vi "信号光谱8.vi"() -> ()   [LabVIEW 2018]
uses:
  <vilib>/Utility/NIReport.llb/Report Type.ctl
  <vilib>/Utility/file.llb/Write Delimited Spreadsheet (DBL).vi
  <vilib>/Instr/_visa.llb/VISA Configure Serial Port (Instr).vi
  <vilib>/addons/_office/excel.llb/Excel Get Data ([str]).vi
  <vilib>/Utility/NIReport.llb/NI_report.lvclass
  <vilib>/Analysis/NI_AALBase.lvlib
  <vilib>/ptbypt/NI_PtbyPt.lvlib
  <vilib>/Utility/NIReport.llb/NI_ReportGenerationCore.lvlib
  <vilib>/addons/_office/NI_ReportGenerationToolkit.lvlib
  <vilib>/Utility/NIReport.llb/Excel/NI_Excel.lvclass
panel:
  in  "上升下降沿/s":dbl format="%.2p"
  in  "延时/s":dbl format="%.2p"
  in  "占空比/%":dbl=3.0 format="%.2p"
  in  "高电平/V":dbl=4.0 format="%.2p"
  in  "频率/Hz":dbl=6000.0 format="%.3p"
  in  "低电平/V":dbl min=0.0 max=5.0 format="%.2p"
  in  "Enable":bool
  in  "上升下降沿":i32(ring)=1 items=["上升沿", "下降沿"]
  in  "输出信号波形":u16(ring) items=["Pulse"]
  out "Output":bool
  in  "VISA 信号发生器":refnum<visa-resource-name>="USB0::0x1AB1::0x0641::DG4E192200870::INSTR"
  out "Output 2":bool
  in  "Enable 2":bool
  in  "上升下降沿/s 2":dbl format="%.2p"
  in  "延时/s 2":dbl format="%.2p"
  in  "占空比/% 2":dbl=3.0 format="%.2p"
  in  "高电平/V 2":dbl=0.002 format="%.2p"
  in  "频率/Hz 2":dbl=6000.0 format="%.3p"
  in  "低电平/V 2":dbl min=0.0 max=5.0 format="%.2p"
  in  "上升下降沿 2":i32(ring)=1 items=["上升沿", "下降沿"]
  in  "输出信号波形 2":u16(ring) items=["Pulse"]
  in  "终止测量":bool
  in  "测量次数":i32=1
  out "best fit":cluster{"Y":dbl[], "Y":dbl[]}[](graph)
  in  "拟合终点":i32=700
  in  "拟合起点":i32=350
  out "angle":dbl
  out "图片地址":string
  in  "开光时间/ms":u32=50
  out "最终存储路径 2":path
  out "照明光error out":errorcluster
  in  "照明光":bool
  in  "stop bits (10: 1 bit)":u16(ring)=10 items=["1.0"=10, "1.5"=15, "2.0"=20]
  in  "parity (0:none)":enum16{"None", "Odd", "Even", "Mark", "Space"}(ring)
  in  "data bits (8)":u16=8 min=5 max=8 step=1
  in  "baud rate":u32=9600 caption="baud rate (115200)" min=9600 max=115200
  in  "照明光VISA":refnum<visa-resource-name>="COM7"
  out "正在测量":bool
  in  "滤波阈值":dbl=1500.0 format="%#_13g"
  out "范围内？":bool[](array[boolean])
  out "w":dbl
  out "xc":dbl
  out "拟合参数":dbl[](array[numeric])
  out "最终存储路径":path
  in  "停止程序":bool
  out "configure error out":errorcluster
  in  "设置参数":bool
  out "output control error  4":errorcluster
  in  "低电平持续输出":bool
  out "output control error  5":errorcluster
  out "output control error":errorcluster
  in  "开始测量":bool
  in  "channel输出口":i32(ring) items=["Channel 1", "Channel 2"]
  out "output control error":errorcluster
  out "Spectrum":cluster{"Y":dbl[], "Y":dbl[]}[](graph)
  out "波长范围":dbl[](array[numeric])
  in  "?":enum32{"IHR 550", "CCD"}(tab)
  in  "Move To\nTarget Positions":bool
  out "Current UniqueID":string="Mono4"
  in  "Mono ID":string(combo)="Mono1"
  in  "Connect":bool
  out "Initialized JY":bool=TRUE
  in  "Force\nInitialization":bool
  in  "Target Grating":string(combo)="2"
  out "Current Description":string="1" caption="Description"
  out "Grating Index":i32=1
  out "Current Grating":dbl=1200.0
  out "Units":string="nm"
  out "Current WL":dbl=897.9988
  out "Exit Mirror\nPosition":i32(ring)=2 items=["EntranceMirror", "ExitMirror", "Front", "Side"]
  out "Entrance Mirror\nPosition":i32(ring)=2 items=["EntranceMirror", "ExitMirror", "Front", "Side"]
  out "Units 2":string="mm"
  out "Front Entrance":dbl
  in  "Target WL":dbl=2670.0
  in  "Exit Mirror":u16(ring)=3 caption="Target Position Exit Mirror" items=["Front"=2, "Side"=3]
  in  "Entrance Mirror":u16(ring)=2 caption="Target Position\nEntrance Mirror" items=["Front"=2, "Side"=3]
  in  "Target\nFront Entrance":dbl=1.0
  in  "Commande tab":T1(tab)
  in  "Area Number to Display":i32
  in  "Reformat":bool
  in  "GAIN":u16(ring)=2 caption="Device Name" items=["High Light", "Best Dynamic Range", "High Sensitivity"]
  in  "ADC":u16(ring) caption="Device Name" items=["20 kHz       ", " 1 MHz       ", " 1 MHz Ultra "]
  in  "Number of Areas :":u16=1 min=1 step=1
  in  "Integration time (ms) :":i16=30000
  out "Uniques ID":u16(ring) items=["CCD1", "CCD2"]
  in  "Device Name":u16(ring) items=["Synapse CCD (Lateral)", "Synapse_IGA (Axial)"]
  in  "Signal type :":enum16{"TTL Rising Edge", "TTL Falling Edge"}(ring)=enum."TTL Falling Edge"
  in  "Trigger Type :":u16(ring) items=["On Start"=1, "Per Acquisition"=2]
  in  "trigSigTypeString":string
  in  "trigEventString":string
  in  "Enable InputTriggers :":bool
  in  "Number of Cleans":i32=1
  in  "MultiAcqShutterMode":i32(ring)=3 items=["Open For All Spectra"=1, "Open for Each Spectrum"=3]
  in  "Accumulations:":u16=10 min=1 step=1
  in  "Multi Accumulation mode:":bool
  out "Y Pixels:":i32=256
  out "DataSize":i32=1024
  out "X Pixels:":i32=1024
  out "Firmware\nVersion":string="V1.20 CCD_4000"
  out "initialized ?":bool=TRUE
  in  "Continuous":bool
  in  "CCD Busy":bool
  out "indicator":string="Ready !"
  in  "initialize":bool
  in  "ShutterOpen":bool=TRUE caption="Shutter enable"
  in  "Acquire":bool
  in  "Temperature":bool
  in  "Setup":bool
  out "Acq Time(ms)":u32=3401
  in  "Save Backlight":bool
  in  "cut backlight":bool
  out "backlight":bool=TRUE
  in  "是否拟合":bool
  in  "是否保存":bool
  in  "Close":bool=TRUE
  out "JYCCDLib.IJYCCDReqd":refnum<k7>
  out "areas :":i32[][](array[numeric])=[[1], [1], [1], [1024], [256], [1], [256]]
  in  "Constante de condition\n(Voir l'aide contextuelle)":bool
  out "temp graph":dbl(graph)=-134.538067
  out "ADC Number":i32[](array[numeric])=[0, 1, 2, 3, 4]
  out "Gain Number":i32[](array[numeric])=[10, 11, 12, 13, 8, 2]
  out "trigAddress":i32
  out "Data":i32[][](graph)
  out "error out":errorcluster
  out "Gratings":dbl[](array[numeric])=[1200.0, 300.0]
  out "Backlight":i32[][](graph)
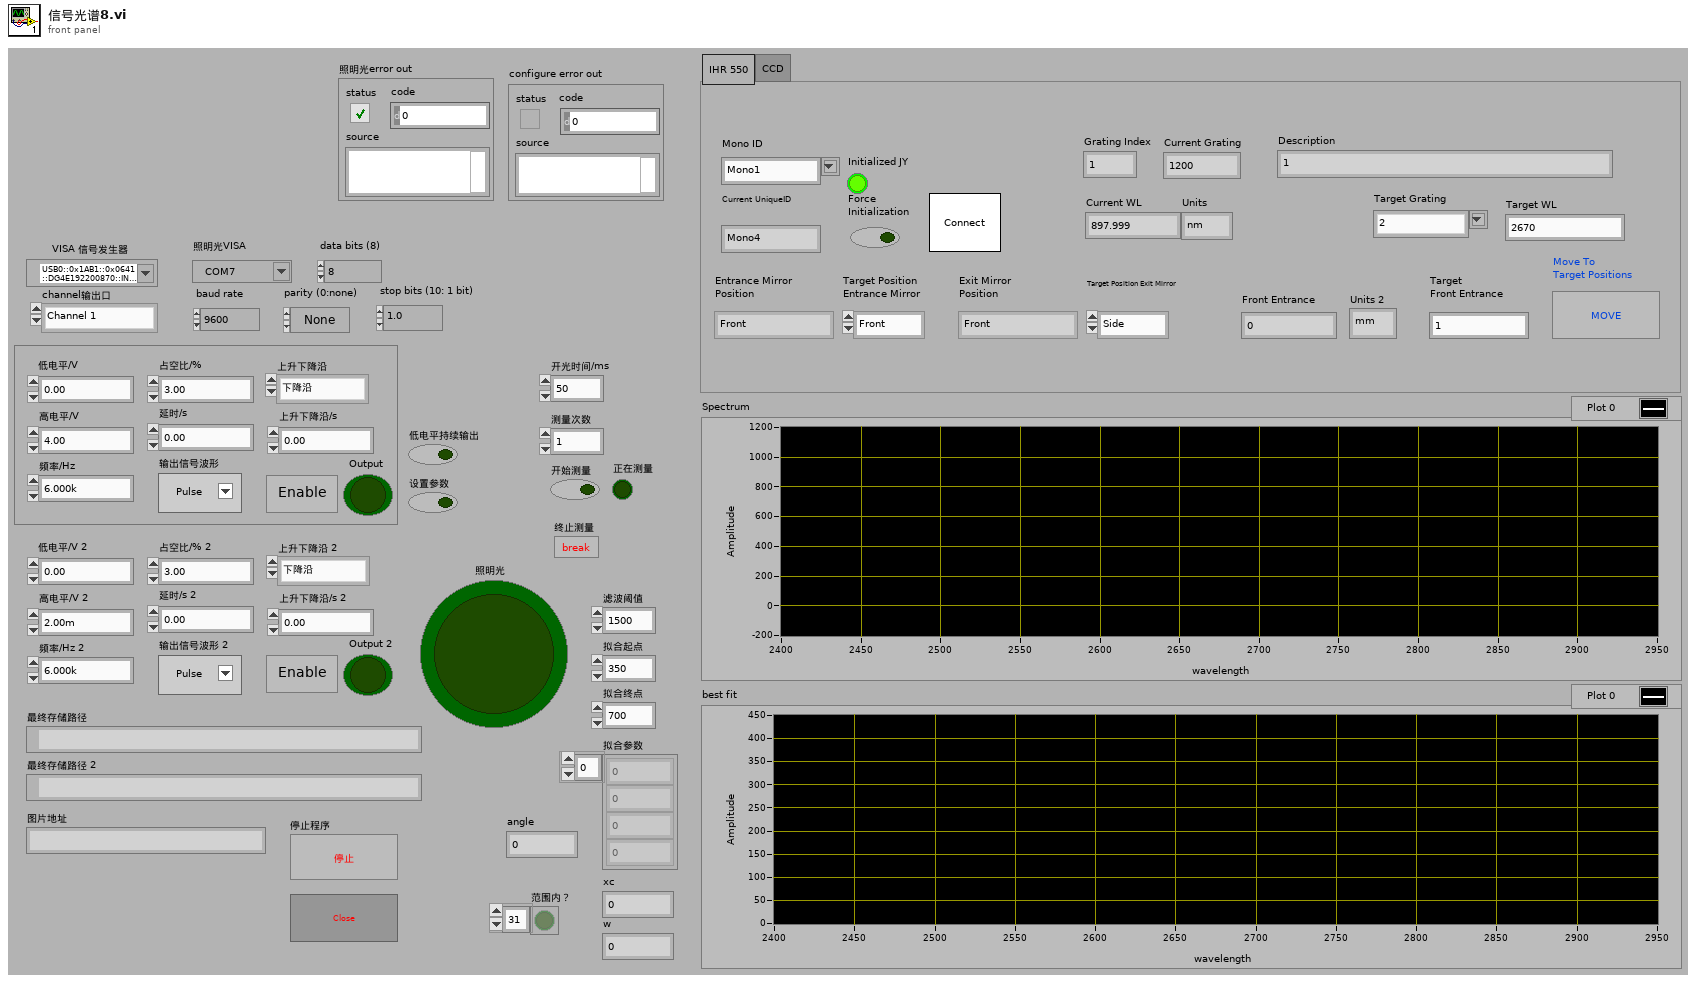
[diagram p1: front panel]
types:
  T1 = enum32{"Settings", "Trigger In", "Multi-Accu.", "Infos"}
  T2 = enum8{"Enabled", "Disabled", "Disabled and Grayed Out"}
  T3 = enum16{"maximized", "minimized", "normal", "no change"}
  T4 = typedef "NI_ReportGenerationCore.lvlib/Report Type.ctl" = enum16{"HTML", "Word", "Excel"}
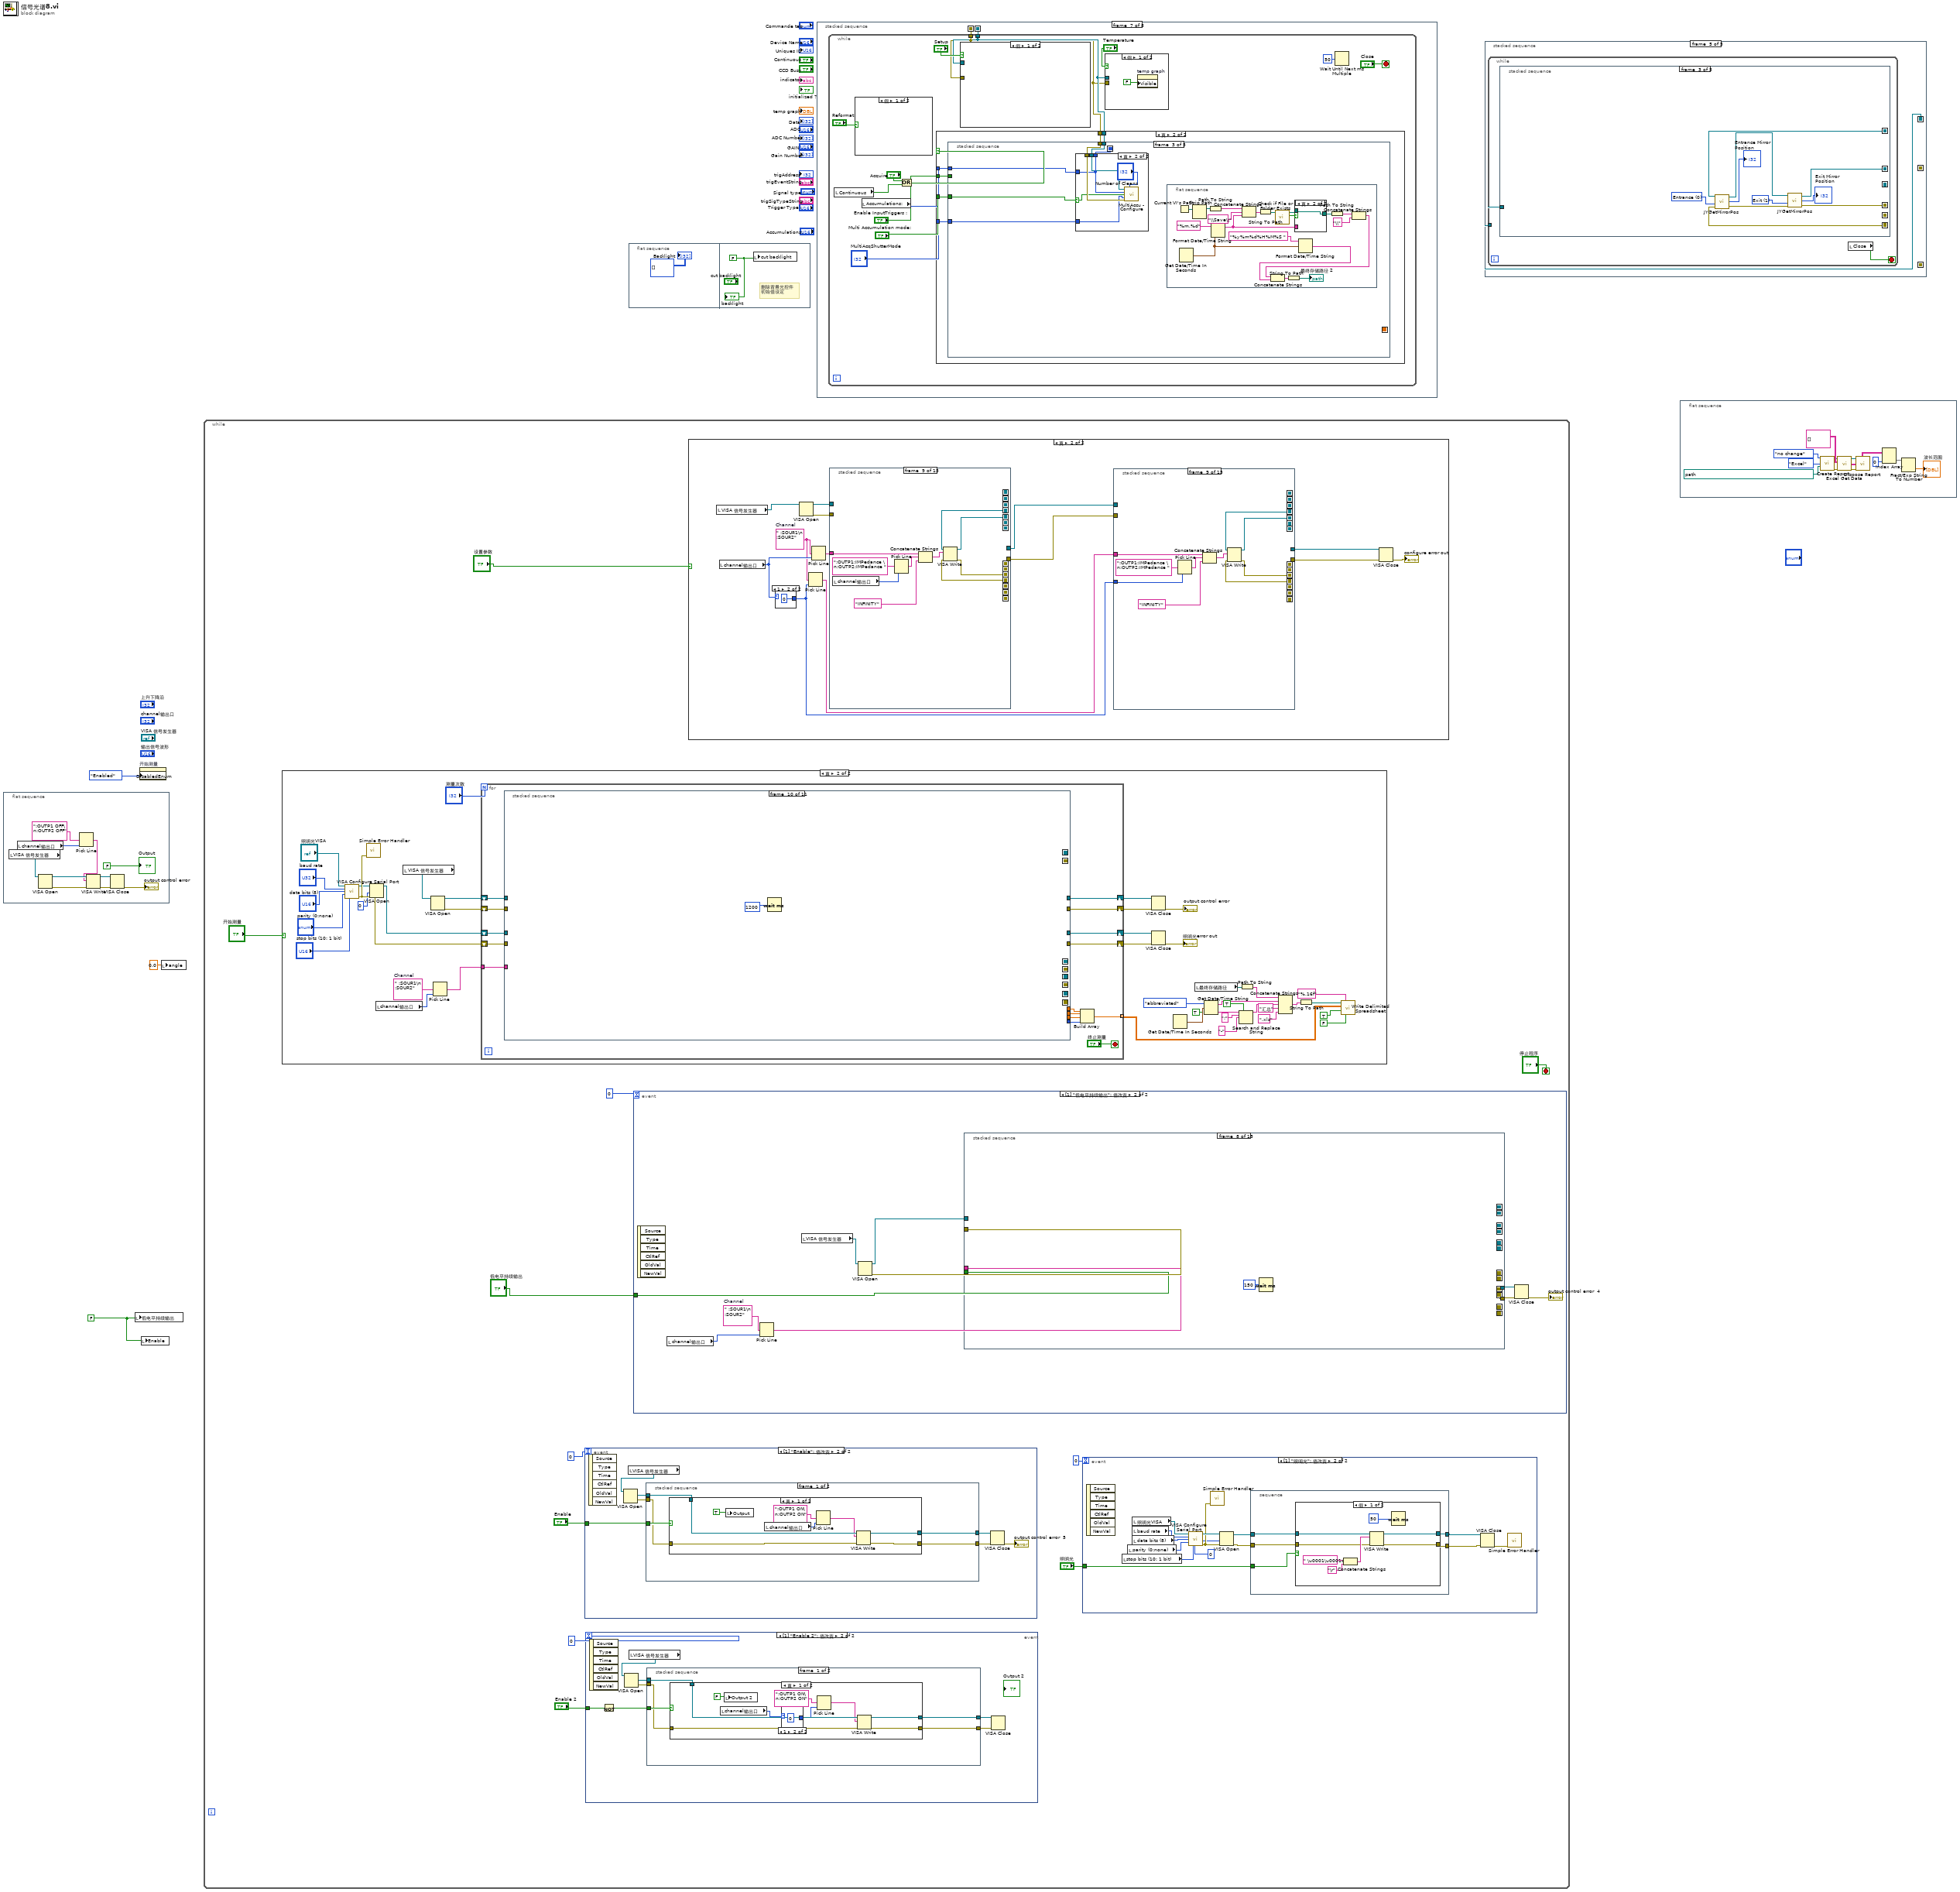
[diagram p0: block diagram]
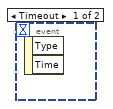
[diagram p2: hidden frame]
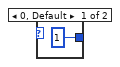
[diagram p3: hidden frame]
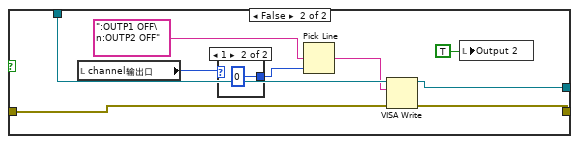
[diagram p4: hidden frame]
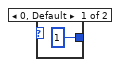
[diagram p5: hidden frame]
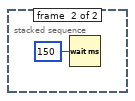
[diagram p6: hidden frame]
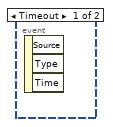
[diagram p7: hidden frame]
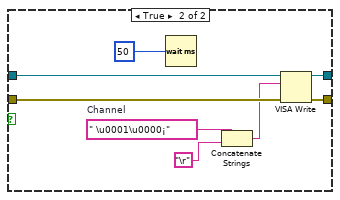
[diagram p8: hidden frame]
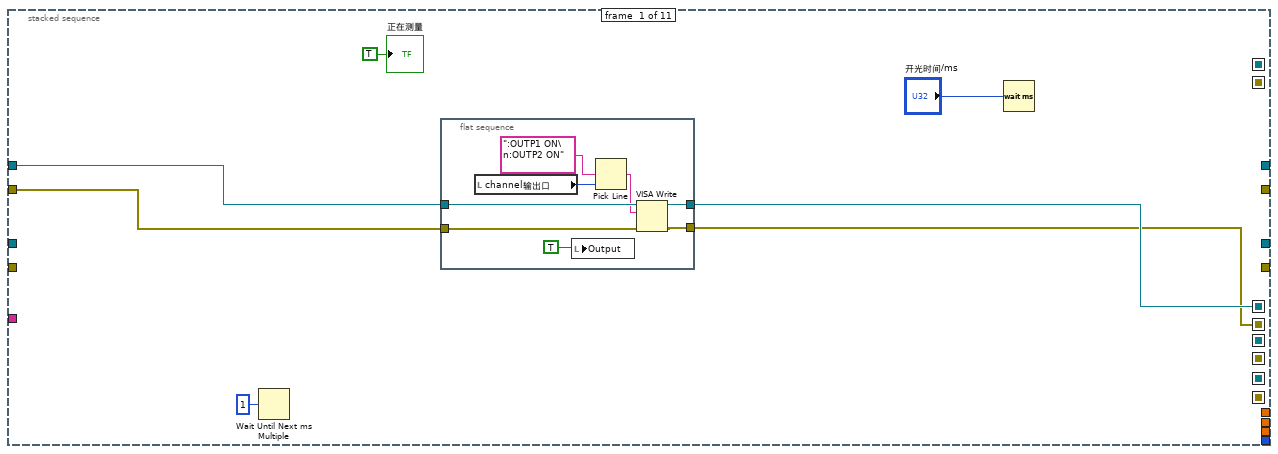
[diagram p10: hidden frame]
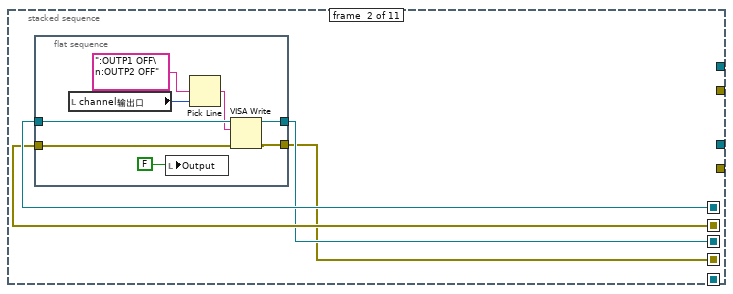
[diagram p11: hidden frame]
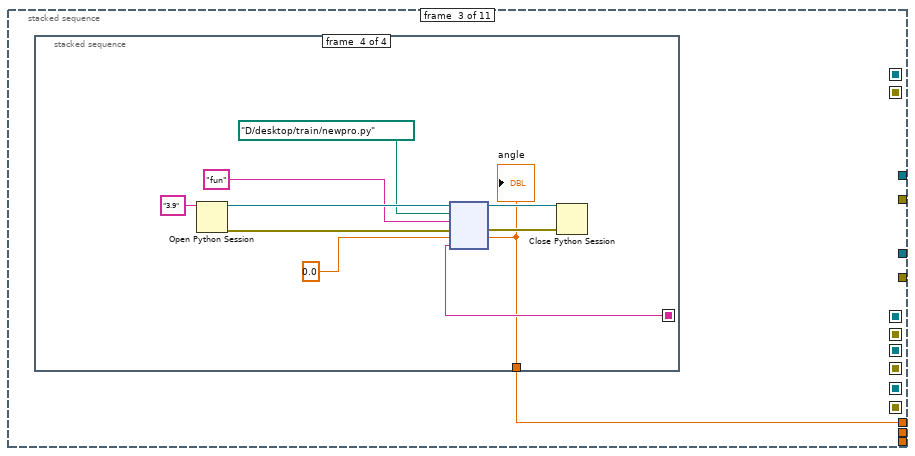
[diagram p12: hidden frame]
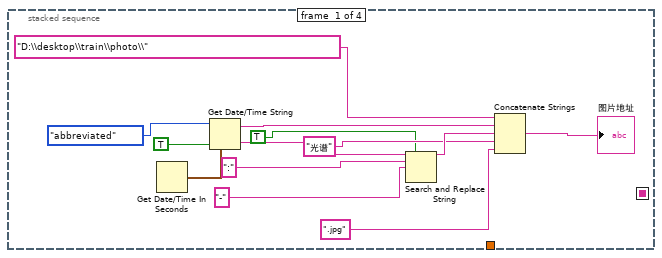
[diagram p13: hidden frame]
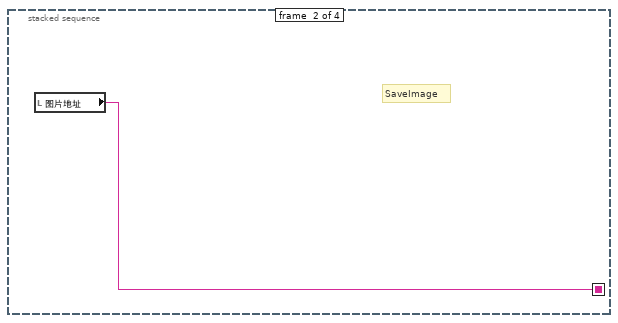
[diagram p14: hidden frame]
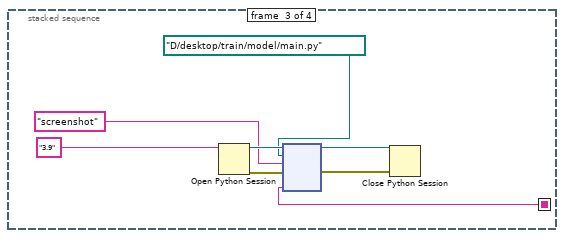
[diagram p15: hidden frame]
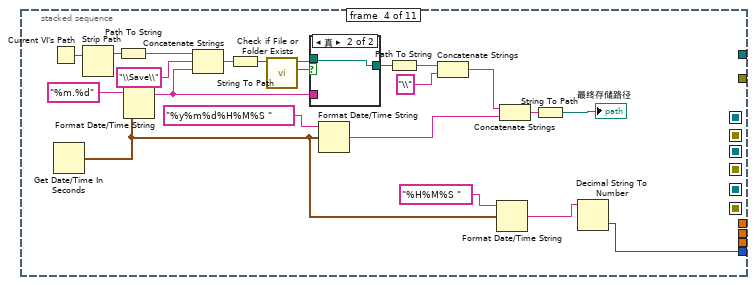
[diagram p16: hidden frame]
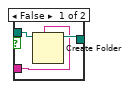
[diagram p17: hidden frame]
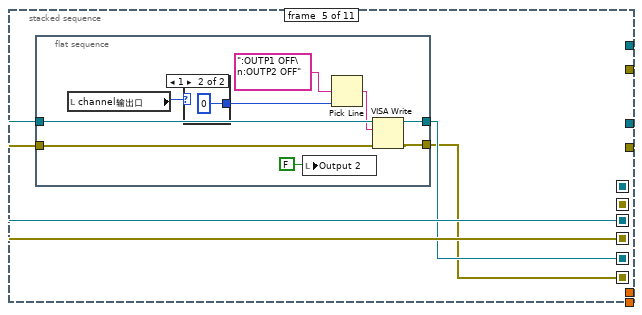
[diagram p18: hidden frame]
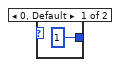
[diagram p19: hidden frame]
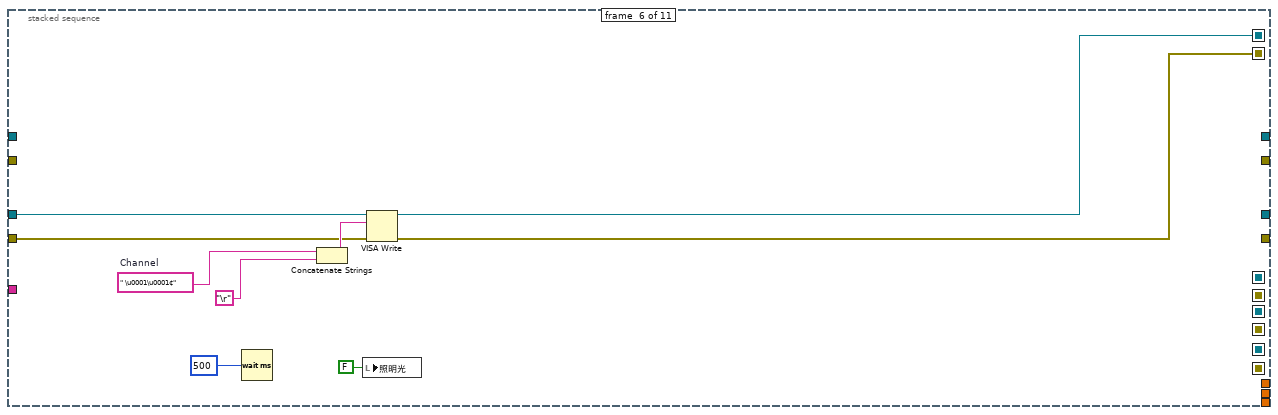
[diagram p20: hidden frame]
diagram:
  w2 = FALSE
  n1 = flat-sequence {
    frame #0 {
      n2 = local read "VISA 信号发生器"() -> (w7:refnum<visa-resource-name>)
      n3 = local read "channel输出口"() -> (w5:i32)
      n4 = VISA Open(VISA resource name=w7) -> (VISA resource name=w13:refnum<visa-resource-name>, error out=w12:errorcluster)  [unwired: 4 in]
      n5 = Pick Line(multi-line string=":OUTP1 OFF\n:OUTP2 OFF" ("write buffer"), line index=w5) -> (output string=w4:string)  [unwired: 1 in]
      n6 = VISA Write(VISA resource name=w13, write buffer=w4, error in (no error)=w12) -> (VISA resource name out=w10:refnum<visa-resource-name>, error out=w9:errorcluster)  [unwired: 1 out]
      n7 = VISA Close(VISA resource name=w10, error in (no error)=w9) -> (error out=→"output control error":errorcluster)
      "Output" <- FALSE ("布尔")
    }
  }
  n8 = local write "低电平持续输出"(w2) -> ()
  n9 = property on="开始测量" class="Bool"("DisabledEnum"=T2."Enabled" ("禁用")) -> ()  [unwired: 2 in, 2 out]
  n10 = local write "Enable"(w2) -> ()
  n11 = local write "angle"(0.0 ("angle")) -> ()
  n12 = while {
    stop <- "停止程序" stop-if-true
    n13 = case shown="真" "开始测量" {
      frame False {
      }
      frame True {
        w130 = " :SOUR1\n :SOUR2"  # Channel
        n14 = call-poly "VISA Configure Serial Port"("VISA resource name"="照明光VISA", "baud rate (9600)"="baud rate", "data bits (8)"="data bits (8)", "parity (0:none)"="parity (0:none)", "stop bits (10: 1 bit)"="stop bits (10: 1 bit)") -> ("VISA resource name out"=w125:refnum<visa-resource-name>, "error out"=w126:errorcluster)  [unwired: 9 in]
        n15 = call <vilib>:"Simple Error Handler.vi"("error in (no error)"=w126) -> ()  [unwired: 4 in, 5 out]
        n16 = VISA Open(access mode=0, error in (no error)=w126, VISA resource name=w125) -> (VISA resource name=w118:refnum<visa-resource-name>, error out=w117:errorcluster)  [unwired: 2 in]
        n17 = local read "channel输出口"() -> (w131:i32)
        n18 = local read "VISA 信号发生器"() -> (w136:refnum<visa-resource-name>)
        n19 = VISA Open(VISA resource name=w136) -> (VISA resource name=w135:refnum<visa-resource-name>, error out=w134:errorcluster)  [unwired: 4 in]
        n20 = Pick Line(multi-line string=w130, line index=w131) -> (output string=w129:string)  [unwired: 1 in]
        n21 = for {
          N: "测量次数" -> [_]
          tunnel: w129 -> [w149]
          shift-right: [w145] -> w128
          shift-left: w135 -> [w151]
          shift-right: [w144] -> w127
          shift-left: w134 -> [w150]
          shift-right: [w143] -> w133
          shift-left: w118 -> [w148]
          shift-right: [w142] -> w132
          shift-left: w117 -> [w147]
          tunnel: [w137] -> w95 mode=indexing
          stop <- "终止测量" stop-if-true
          n22 = stacked-sequence {
            seq-local: [w153 _ _ _ _ _ _ _ _ _ _] -> [_ w170 _ _ _ _ _ _ _ _ _]
            seq-local: [w152 _ _ _ _ _ _ _ _ _ _] -> [_ w169 _ _ _ _ _ _ _ _ _]
            seq-local: [_ _ _ _ _ w255 _ _ _ _ _] -> [_ _ _ _ _ _ _ _ w370 _ _]
            seq-local: [_ _ _ _ _ w254 _ _ _ _ _] -> [_ _ _ _ _ _ _ _ w373 _ _]
            seq-local: [_ w168 _ _ _ _ _ _ _ _ _] -> [_ _ _ _ w241 _ _ _ _ _ _]
            seq-local: [_ w167 _ _ _ _ _ _ _ _ _] -> [_ _ _ _ w240 _ _ _ _ _ _]
            seq-local: [_ _ _ _ w239 _ _ _ _ _ _] -> [_ _ _ _ _ _ _ w356 _ _ _]
            seq-local: [_ _ _ _ w238 _ _ _ _ _ _] -> [_ _ _ _ _ _ _ w355 _ _ _]
            tunnel: w151 -> [w155 _ _ _ _ _ _ _ _ _ _]
            tunnel: w150 -> [w154 _ _ _ _ _ _ _ _ _ _]
            tunnel: [_ _ _ _ _ _ _ w354 _ _ _] -> w145
            tunnel: [_ _ _ _ _ _ _ w353 _ _ _] -> w144
            tunnel: w149 -> [_ _ _ _ _ _ _ _ _ _ _]
            tunnel: w148 -> [_ _ _ _ _ w258 _ _ _ _ _]
            tunnel: w147 -> [_ _ _ _ _ w257 _ _ _ _ _]
            tunnel: [_ _ _ _ _ _ _ _ w372 _ _] -> w143
            tunnel: [_ _ _ _ _ _ _ _ w371 _ _] -> w142
            tunnel: [_ _ w179 _ _ _ _ _ _ _ _] -> w141
            tunnel: [_ _ _ _ _ _ w263 _ _ _ _] -> w140
            tunnel: [_ _ _ _ _ _ w262 _ _ _ _] -> w139
            tunnel: [_ _ _ w212 _ _ _ _ _ _ _] -> w138
            frame #0 {
              n23 = Wait Until Next ms Multiple(millisecond multiple=u32 1 ("毫秒倍数")) -> ()  [unwired: 1 out]
              n24 = flat-sequence {
                tunnel: w155 -> [w166]
                tunnel: w154 -> [w165]
                tunnel: [w160] -> w153
                tunnel: [w159] -> w152
                frame #0 {
                  n25 = local read "channel输出口"() -> (w162:i32)
                  n26 = local write "Output"(TRUE ("布尔")) -> ()
                  n27 = Pick Line(multi-line string=":OUTP1 ON\n:OUTP2 ON" ("write buffer"), line index=w162) -> (output string=w161:string)  [unwired: 1 in]
                  n28 = VISA Write(VISA resource name=w166, write buffer=w161, error in (no error)=w165) -> (VISA resource name out=w160:refnum<visa-resource-name>, error out=w159:errorcluster)  [unwired: 1 out]
                }
              }
              n29 = Wait (ms)(milliseconds to wait="开光时间/ms") -> ()  [unwired: 1 out]
              "正在测量" <- TRUE
            }
            frame #1 {
              n30 = flat-sequence {
                tunnel: w170 -> [w178]
                tunnel: w169 -> [w177]
                tunnel: [w172] -> w168
                tunnel: [w171] -> w167
                frame #0 {
                  n31 = local read "channel输出口"() -> (w174:i32)
                  n32 = local write "Output"(FALSE ("布尔")) -> ()
                  n33 = Pick Line(multi-line string=":OUTP1 OFF\n:OUTP2 OFF" ("write buffer"), line index=w174) -> (output string=w173:string)  [unwired: 1 in]
                  n34 = VISA Write(VISA resource name=w178, write buffer=w173, error in (no error)=w177) -> (VISA resource name out=w172:refnum<visa-resource-name>, error out=w171:errorcluster)  [unwired: 1 out]
                }
              }
            }
            frame #2 {
              n35 = stacked-sequence {
                seq-local: [_ w193 _ _] -> [_ _ w194 w203]
                tunnel: [_ _ _ w202] -> w179
                frame #0 {
                  n36 = Get Date/Time In Seconds() -> (seconds since 1Jan1904=w189:timestamp)
                  n37 = Get Date/Time String(date format (0)=enum16{"short", "long", "abbreviated"}."abbreviated" ("日期格式(0)"), seconds (now)=w189, want seconds? (F)=TRUE ("需要秒？(F)")) -> (date string=w192:string, time string=w190:string)
                  n38 = Search and Replace String(replace all?=TRUE ("替换全部？(F)"), input string=w190, search string=":" ("搜索字符串"), replace string="-" ("替换字符串(\"\")")) -> (result string=w191:string)  [unwired: 4 in, 3 out]
                  n39 = Concatenate Strings("D:\\desktop\\train\\photo\\", w192, w191, "光谱" ("字符串"), ".jpg" ("字符串")) -> (→"图片地址":string)
                }
                frame #1 {
                  # "SaveImage"
                  n40 = local read "图片地址"() -> (w193:string)
                }
                frame #2 {
                  n41 = Open Python Session(python version="3.9" ("Python version")) -> (session out=w201:refnum<k35>, error out=w199:errorcluster)  [unwired: 2 in]
                  n42 = node(w201, path "D:/desktop/train/model/main.py" ("module path"), "screenshot" ("function name"), w199, w194) -> (w200:refnum<k35>, w198:errorcluster)  [unwired: 3 in, 2 out]
                  n43 = Close Python Session(session in=w200, error in=w198) -> ()  [unwired: 1 out]
                }
                frame #3 {
                  n44 = Open Python Session(python version="3.9" ("Python version")) -> (session out=w210:refnum<k35>, error out=w208:errorcluster)  [unwired: 2 in]
                  n45 = node(w210, path "D:/desktop/train/newpro.py" ("module path"), "fun" ("function name"), w208, 0.0, w203) -> (w209:refnum<k35>, w207:errorcluster, w202:dbl)  [unwired: 1 in, 2 out]
                  "angle" <- w202
                  n46 = Close Python Session(session in=w209, error in=w207) -> ()  [unwired: 1 out]
                }
              }
            }
            frame #3 {
              n47 = Current VI's Path() -> (path=w221:path)
              n48 = Get Date/Time In Seconds() -> (seconds since 1Jan1904=w214:timestamp)
              n49 = Strip Path(path=w221) -> (stripped path=w222:path)  [unwired: 1 out]
              n50 = Path To String(path=w222) -> (string=w223:string)
              n51 = Format Date/Time String(time format string (%c)="%m.%d" ("时间格式字符串(%c)"), seconds (now)=w214) -> (date/time string=w229:string)  [unwired: 1 in]
              n52 = Concatenate Strings(w223, "\\Save\\" ("字符串"), w229) -> (w224:string)
              n53 = String To Path(string=w224) -> (path=w225:path)
              n54 = call <vilib>:"Check if File or Folder Exists.vi"("path"=w225) -> ("file or folder exists?"=w226:bool, "dup path"=w228:path)  [unwired: 8 in, 1 out]
              n55 = case shown="真" w226 {
                tunnel: [w236 w237] -> w227
                tunnel: w228 -> [w235 w237]
                tunnel: w229 -> [w234 _]
                frame False {
                  n56 = Create Folder(prompt (Create Folder)=w234, path (use dialog)=w235) -> (created path=w236:path)  [unwired: 1 in, 2 out]
                }
                frame True {
                }
              }
              n57 = Format Date/Time String(time format string (%c)="%y%m%d%H%M%S " ("时间格式字符串(%c)"), seconds (now)=w214) -> (date/time string=w232:string)  [unwired: 1 in]
              n58 = Path To String(path=w227) -> (string=w230:string)
              n59 = Concatenate Strings(w230, "\\" ("字符串")) -> (w231:string)
              n60 = Format Date/Time String(time format string (%c)="%H%M%S " ("时间格式字符串(%c)"), seconds (now)=w214) -> (date/time string=w213:string)  [unwired: 1 in]
              n61 = Concatenate Strings(w231, w232) -> (w220:string)
              n62 = String To Path(string=w220) -> (path=→"最终存储路径":path)
              n63 = Decimal String To Number(string=w213) -> (number=w212:i32)  [unwired: 2 in, 1 out]
            }
            frame #4 {
              n64 = flat-sequence {
                tunnel: w241 -> [w250]
                tunnel: w240 -> [w249]
                tunnel: [w245] -> w239
                tunnel: [w244] -> w238
                frame #0 {
                  n65 = local read "channel输出口"() -> (w243:i32)
                  n66 = case shown="1" w243 {
                    tunnel: [1 0] -> w242
                    frame 0, Default {
                    }
                    frame 1 {
                    }
                  }
                  n67 = local write "Output 2"(FALSE ("布尔")) -> ()
                  n68 = Pick Line(multi-line string=":OUTP1 OFF\n:OUTP2 OFF" ("write buffer"), line index=w242) -> (output string=w246:string)  [unwired: 1 in]
                  n69 = VISA Write(VISA resource name=w250, write buffer=w246, error in (no error)=w249) -> (VISA resource name out=w245:refnum<visa-resource-name>, error out=w244:errorcluster)  [unwired: 1 out]
                }
              }
            }
            frame #5 {
              w253 = " \u0001\u0001¢"  # Channel
              n70 = Wait (ms)(milliseconds to wait=500) -> ()  [unwired: 1 out]
              n71 = Concatenate Strings(w253, "\r") -> (w259:string)
              n72 = local write "照明光"(FALSE ("照明光")) -> ()
              n73 = VISA Write(VISA resource name=w258, write buffer=w259, error in (no error)=w257) -> (VISA resource name out=w255:refnum<visa-resource-name>, error out=w254:errorcluster)  [unwired: 1 out]
            }
            frame #6 {
              n74 = local read "Area Number to Display"() -> (w306:i32)
              n75 = local read "JYCCDLib.IJYCCDReqd"() -> (w302:refnum<k7>)
              n76 = Get Date/Time In Seconds() -> (seconds since 1Jan1904=w315:timestamp)
              n77 = local read "最终存储路径"() -> (w329:path)
              n78 = Get Date/Time String(date format (0)=enum16{"short", "long", "abbreviated"}."abbreviated" ("日期格式(0)"), seconds (now)=w315, want seconds? (F)=TRUE ("需要秒？(F)")) -> (date string=w323:string, time string=w318:string)
              n79 = call "MultiAccu - Acquire spectral.vi"("error in"=errorcluster {"status"=FALSE, "code"=0, "source"=""}, "Accumulations:"=u16 1, "ShutterOpen"=TRUE, "JYCCDLib.IJYCCDReqd"=w302) -> ("Acq Time(ms)"=w308:u32, "Array Out"=w307:i32[][][])  [unwired: 1 out]
              n80 = local write "Acq Time(ms)"(w308) -> ()
              n81 = local read "cut backlight"() -> (w290:bool)
              n82 = local read "backlight"() -> (w288:bool)
              n83 = Search and Replace String(replace all?=TRUE ("替换全部？(F)"), input string=w318, search string=":" ("搜索字符串"), replace string="-" ("替换字符串(\"\")")) -> (result string=w322:string)  [unwired: 4 in, 3 out]
              n84 = Path To String(path=w329) -> (string=w312:string)
              n85 = And(x=w290, y=w288) -> (x .and. y?=w289:bool)
              n86 = call "Array reset dimension.vi"("Area Number"=w306, "Array In"=w307) -> ("Array Out"=w292:i32[][])
              n87 = Concatenate Strings(w312, w323, w322, "光谱" ("字符串"), ".xls" ("字符串")) -> (w327:string)
              n88 = case shown="真" w289 {
                tunnel: [w349 w351] -> w291
                tunnel: w292 -> [w349 w350]
                frame False {
                }
                frame True {
                  n89 = local read "Backlight"() -> (w352:i32[][])
                  n90 = Subtract(x=w350, y=w352) -> (x-y=w351:i32[][])
                }
              }
              n91 = String To Path(string=w327) -> (path=w328:path)
              n92 = local write "Data"(w292) -> ()
              n93 = local read "波长范围"() -> (w269:dbl[])
              n94 = Index Array(array=w291, index (row)=0 ("索引 (行)")) -> (element=w330:i32[])  [unwired: 1 in]
              n95 = Reverse 1D Array(array=w330) -> (reversed array=w265:i32[])
              n96 = local read "angle"() -> (w268:dbl)
              n97 = local read "拟合起点"() -> (w278:i32)
              n98 = local read "拟合终点"() -> (w280:i32)
              n99 = call <vilib>:"Median Filter.vi"("left rank"=6, "X"=w265) -> ("Filtered X"=w264:dbl[])  [unwired: 8 in, 1 out]
              n100 = Build Array(w268, 0.0 ("元素")) -> (w266:dbl[])
              n101 = Subtract(x=w280, y=w278) -> (x-y=w277:i32)
              n102 = call "Convert to Dynamic Data"("Array"=w269) -> ("Dynamic Data Type"=w299:dynamicdata)  [unwired: 3 in]
              n103 = call "Convert to Dynamic Data2"("Array"=w265) -> ("Dynamic Data Type"=w298:dynamicdata)  [unwired: 3 in]
              n104 = Array Subset(array=w269, index=w278, length=w277) -> (w275:dbl[])
              n105 = call "Build XY Graph"("Y Input"=w298, "X Input"=w299) -> ("XY Graph"=→"Spectrum":cluster{"Y":dbl[], "Y":dbl[]}[])  [unwired: 8 in, 1 out]
              n106 = call "转换至动态数据4"("Array"=w275) -> ("Dynamic Data Type"=w296:dynamicdata)  [unwired: 3 in]
              n107 = In Range and Coerce(upper limit="滤波阈值", x=w264, lower limit=-100.0) -> (In Range?=w283:bool[])  [unwired: 1 out]
              "范围内？" <- w283
              n108 = Not(x=w283) -> (.not. x?=w282:bool[])
              n109 = Or Array Elements(Boolean array=w282) -> (logical OR=w285:bool)
              n110 = local read "X Pixels:"() -> (w284:i32)
              n111 = local read "波长范围"() -> (w270:dbl[])
              n112 = local read "滤波阈值"() -> (w281:dbl)
              n113 = case shown="真" w285 {
                tunnel: w284 -> [_ w336]
                tunnel: w264 -> [w332 w335]
                tunnel: [w332 w334] -> w276
                tunnel: w281 -> [_ w333]
                frame False {
                }
                frame True {
                  n114 = for {
                    N: w336 -> [_]
                    tunnel: w335 -> [w340] mode=indexing
                    tunnel: [w339] -> w334 mode=indexing
                    shift-right: [w339] -> _
                    shift-left: _ -> [w338]
                    tunnel: w333 -> [w337]
                    n115 = Greater?(x=w340, y=w337) -> (0:w342:bool)
                    n116 = Less?(x=w340, y=-100.0) -> (x < y?=w343:bool)
                    n117 = Or(x=w342, y=w343) -> (x .or. y?=w341:bool)
                    n118 = case shown="真" w341 {
                      tunnel: w340 -> [w345 _]
                      tunnel: [w345 w347] -> w339
                      tunnel: w338 -> [_ w348]
                      frame False {
                      }
                      frame True {
                        n119 = call <vilib>:"Median Filter PtByPt.vi"("rank"=5, "x"=w348) -> ("Filtered x"=w347:dbl)  [unwired: 2 in, 1 out]
                      }
                    }
                  }
                }
              }
              n120 = Array Subset(array=w276, index=w278, length=w277) -> (w279:dbl[])
              n121 = call "转换至动态数据3"("Array"=w279) -> ("Dynamic Data Type"=w297:dynamicdata)  [unwired: 3 in]
              n122 = call "曲线拟合"("Locations"=w296, "Signals"=w297) -> ("best fit"=w301:dynamicdata, "non-linear coefficients"=w300:dynamicdata)  [unwired: 5 in, 3 out]
              n123 = call "从动态数据转换"("Dynamic Data Type"=w300) -> ("Array"=w293:dbl[])  [unwired: 3 in]
              "拟合参数" <- w293
              n124 = call "从动态数据转换2"("Dynamic Data Type"=w301) -> ("Array"=w274:dbl[])  [unwired: 3 in]
              n125 = Build Array(w269, w264, w274, w293, w266) -> (w331:dbl[][])
              n126 = call-poly <vilib>:"Write Delimited Spreadsheet.vi"("file path (dialog if empty)"=w328, "format (%.3f)"="%.16f", "2D data"=w331, "append to file? (new file:F)"=TRUE ("append to file? (F)"), "transpose? (no:F)"=TRUE ("transpose? (F)")) -> ()  [unwired: 9 in, 2 out]
              n127 = Index Array(array=w293, index #1=0 ("索引"), index #2=1 ("索引")) -> (element #1=w263:dbl, element #2=w262:dbl)
              "xc" <- w263
              "w" <- w262
              n128 = Bundle("波长范围"=w270, "Filtered X"=w276) -> (w273:cluster{"波长范围 ":dbl[], "Filtered X":dbl[]})  [unwired: 1 in]
              n129 = Bundle(w275, "Array"=w274) -> (w272:cluster{dbl[], "Array":dbl[]})  [unwired: 1 in]
              n130 = Build Array(w273, w272) -> (w271:cluster{"波长范围 ":dbl[], "Array":dbl[]}[])
              n131 = local write "best fit"(w271) -> ()
            }
            frame #7 {
              n132 = flat-sequence {
                tunnel: w356 -> [w365]
                tunnel: w355 -> [w364]
                tunnel: [w360] -> w354
                tunnel: [w359] -> w353
                frame #0 {
                  n133 = local read "channel输出口"() -> (w358:i32)
                  n134 = case shown="1" w358 {
                    tunnel: [1 0] -> w357
                    frame 0, Default {
                    }
                    frame 1 {
                    }
                  }
                  n135 = local write "Output 2"(TRUE ("布尔")) -> ()
                  n136 = Pick Line(multi-line string=":OUTP1 ON\n:OUTP2 ON" ("write buffer"), line index=w357) -> (output string=w361:string)  [unwired: 1 in]
                  n137 = VISA Write(VISA resource name=w365, write buffer=w361, error in (no error)=w364) -> (VISA resource name out=w360:refnum<visa-resource-name>, error out=w359:errorcluster)  [unwired: 1 out]
                }
              }
            }
            frame #8 {
              w368 = " \u0001\u0000¡"  # Channel
              n138 = Concatenate Strings(w368, "\r") -> (w374:string)
              n139 = VISA Write(VISA resource name=w370, write buffer=w374, error in (no error)=w373) -> (VISA resource name out=w372:refnum<visa-resource-name>, error out=w371:errorcluster)  [unwired: 1 out]
              n140 = local write "照明光"(TRUE ("照明光")) -> ()
            }
            frame #9 {
              n141 = Wait (ms)(milliseconds to wait=1200) -> ()  [unwired: 1 out]
            }
            frame #10 {
              n142 = local write "正在测量"(FALSE) -> ()
            }
          }
          n143 = Build Array(w141, w140, w139, w138) -> (w137:dbl[])
        }
        n144 = VISA Close(VISA resource name=w128, error in (no error)=w127) -> (error out=→"output control error":errorcluster)
        n145 = VISA Close(VISA resource name=w133, error in (no error)=w132) -> (error out=→"照明光error out":errorcluster)
        n146 = Get Date/Time In Seconds() -> (seconds since 1Jan1904=w112:timestamp)
        n147 = local read "最终存储路径"() -> (w106:path)
        n148 = Get Date/Time String(date format (0)=enum16{"short", "long", "abbreviated"}."abbreviated" ("日期格式(0)"), seconds (now)=w112, want seconds? (F)=TRUE ("需要秒？(F)")) -> (date string=w109:string, time string=w111:string)
        n149 = Search and Replace String(replace all?=TRUE ("替换全部？(F)"), input string=w111, search string=":" ("搜索字符串"), replace string="-" ("替换字符串(\"\")")) -> (result string=w110:string)  [unwired: 4 in, 3 out]
        n150 = Path To String(path=w106) -> (string=w113:string)
        n151 = Concatenate Strings(w113, w109, w110, "汇总" ("字符串"), ".xls" ("字符串")) -> (w108:string)
        n152 = String To Path(string=w108) -> (path=w107:path)
        n153 = call-poly <vilib>:"Write Delimited Spreadsheet.vi"("file path (dialog if empty)"=w107, "format (%.3f)"="%.16f", "2D data"=w95, "append to file? (new file:F)"=TRUE ("append to file? (F)"), "transpose? (no:F)"=FALSE ("transpose? (F)")) -> ()  [unwired: 9 in, 2 out]
      }
    }
    n154 = event shown="[1] \"Enable\": 值改变" {
      selector: _ -> [_ _]
      dyn-events: _ -> [_ _]
      timeout: u32 0 ("Time") -> [_ _]
      tunnel: "Enable" -> [_ w382]
      event Timeout {
        n155 = event-data() -> ()  [unwired: 1 in, 2 out]
      }
      event "Enable": Value Change {
        n156 = event-data() -> ()  [unwired: 1 in, 6 out]
        n157 = local read "VISA 信号发生器"() -> (w378:refnum<visa-resource-name>)
        n158 = VISA Open(VISA resource name=w378) -> (VISA resource name=w381:refnum<visa-resource-name>, error out=w384:errorcluster)  [unwired: 4 in]
        n159 = stacked-sequence {
          tunnel: w382 -> [w389 _]
          tunnel: w384 -> [w388 _]
          tunnel: w381 -> [w387 _]
          tunnel: [w386 _] -> w380
          tunnel: [w385 _] -> w379
          frame #0 {
            n160 = case shown="真" w389 {
              tunnel: w387 -> [w397 w405]
              tunnel: [w396 w404] -> w385
              tunnel: w388 -> [w395 w402]
              tunnel: [w394 w403] -> w386
              frame True {
                n161 = local write "Output"(TRUE ("布尔")) -> ()
                n162 = local read "channel输出口"() -> (w391:i32)
                n163 = Pick Line(multi-line string=":OUTP1 ON\n:OUTP2 ON" ("write buffer"), line index=w391) -> (output string=w390:string)  [unwired: 1 in]
                n164 = VISA Write(VISA resource name=w397, write buffer=w390, error in (no error)=w395) -> (VISA resource name out=w394:refnum<visa-resource-name>, error out=w396:errorcluster)  [unwired: 1 out]
              }
              frame False {
                n165 = local read "channel输出口"() -> (w399:i32)
                n166 = Pick Line(multi-line string=":OUTP1 OFF\n:OUTP2 OFF" ("write buffer"), line index=w399) -> (output string=w398:string)  [unwired: 1 in]
                n167 = VISA Write(VISA resource name=w405, write buffer=w398, error in (no error)=w402) -> (VISA resource name out=w403:refnum<visa-resource-name>, error out=w404:errorcluster)  [unwired: 1 out]
                n168 = local write "Output"(FALSE ("布尔")) -> ()
              }
            }
          }
          frame #1 {
            n169 = Wait (ms)(milliseconds to wait=u32 150) -> ()  [unwired: 1 out]
          }
        }
        n170 = VISA Close(VISA resource name=w380, error in (no error)=w379) -> (error out=→"output control error  5":errorcluster)
      }
    }
    n171 = event shown="[1] \"Enable 2\": 值改变" {
      selector: _ -> [_ _]
      dyn-events: _ -> [_ _]
      timeout: u32 0 ("Time") -> [_ _]
      tunnel: "Enable 2" -> [_ w26]
      event Timeout {
        n172 = event-data() -> ()  [unwired: 1 in, 2 out]
      }
      event "Enable 2": Value Change {
        n173 = event-data() -> ()  [unwired: 1 in, 6 out]
        n174 = Not(x=w26) -> (.not. x?=w25:bool)
        n175 = local read "VISA 信号发生器"() -> (w27:refnum<visa-resource-name>)
        n176 = VISA Open(VISA resource name=w27) -> (VISA resource name=w30:refnum<visa-resource-name>, error out=w31:errorcluster)  [unwired: 4 in]
        n177 = stacked-sequence {
          tunnel: w25 -> [w36 _]
          tunnel: w31 -> [w35 _]
          tunnel: w30 -> [w34 _]
          tunnel: [w33 _] -> w29
          tunnel: [w32 _] -> w28
          frame #0 {
            n178 = case shown="真" w36 {
              tunnel: w34 -> [w45 w56]
              tunnel: [w44 w55] -> w32
              tunnel: w35 -> [w43 w53]
              tunnel: [w42 w54] -> w33
              frame True {
                n179 = local read "channel输出口"() -> (w38:i32)
                n180 = local write "Output 2"(FALSE ("布尔")) -> ()
                n181 = case shown="1" w38 {
                  tunnel: [1 0] -> w37
                  frame 0, Default {
                  }
                  frame 1 {
                  }
                }
                n182 = Pick Line(multi-line string=":OUTP1 ON\n:OUTP2 ON" ("write buffer"), line index=w37) -> (output string=w39:string)  [unwired: 1 in]
                n183 = VISA Write(VISA resource name=w45, write buffer=w39, error in (no error)=w43) -> (VISA resource name out=w42:refnum<visa-resource-name>, error out=w44:errorcluster)  [unwired: 1 out]
              }
              frame False {
                n184 = local read "channel输出口"() -> (w49:i32)
                n185 = case shown="1" w49 {
                  tunnel: [1 0] -> w48
                  frame 0, Default {
                  }
                  frame 1 {
                  }
                }
                n186 = Pick Line(multi-line string=":OUTP1 OFF\n:OUTP2 OFF" ("write buffer"), line index=w48) -> (output string=w50:string)  [unwired: 1 in]
                n187 = VISA Write(VISA resource name=w56, write buffer=w50, error in (no error)=w53) -> (VISA resource name out=w54:refnum<visa-resource-name>, error out=w55:errorcluster)  [unwired: 1 out]
                n188 = local write "Output 2"(TRUE ("布尔")) -> ()
              }
            }
          }
          frame #1 {
            n189 = Wait (ms)(milliseconds to wait=u32 150) -> ()  [unwired: 1 out]
          }
        }
        n190 = VISA Close(VISA resource name=w29, error in (no error)=w28) -> ()  [unwired: 1 out]
      }
    }
    n191 = event shown="[1] \"低电平持续输出\": 值改变" {
      selector: _ -> [_ _]
      dyn-events: _ -> [_ _]
      timeout: u32 0 ("Time") -> [_ _]
      tunnel: "低电平持续输出" -> [_ w407]
      event Timeout {
        n192 = event-data() -> ()  [unwired: 1 in, 2 out]
      }
      event "低电平持续输出": Value Change {
        w411 = " :SOUR1\n :SOUR2"  # Channel
        n193 = event-data() -> ()  [unwired: 1 in, 6 out]
        n194 = local read "channel输出口"() -> (w412:i32)
        n195 = Pick Line(multi-line string=w411, line index=w412) -> (output string=w410:string)  [unwired: 1 in]
        n196 = local read "VISA 信号发生器"() -> (w415:refnum<visa-resource-name>)
        n197 = VISA Open(VISA resource name=w415) -> (VISA resource name=w414:refnum<visa-resource-name>, error out=w413:errorcluster)  [unwired: 4 in]
        n198 = stacked-sequence {
          seq-local: [w421 _ _ _ _ _ _ _ _ _ _ _ _] -> [_ _ w436 _ _ _ _ _ _ _ _ _ _]
          seq-local: [w420 _ _ _ _ _ _ _ _ _ _ _ _] -> [_ _ w435 _ _ _ _ _ _ _ _ _ _]
          seq-local: [_ _ w434 _ _ _ _ _ _ _ _ _ _] -> [_ _ _ _ w439 _ _ _ _ _ _ _ _]
          seq-local: [_ _ w433 _ _ _ _ _ _ _ _ _ _] -> [_ _ _ _ w440 _ _ _ _ _ _ _ _]
          seq-local: [_ _ _ _ w448 _ _ _ _ _ _ _ _] -> [_ _ _ _ _ _ w459 _ _ _ _ _ _]
          seq-local: [_ _ _ _ w447 _ _ _ _ _ _ _ _] -> [_ _ _ _ _ _ w458 _ _ _ _ _ _]
          seq-local: [_ _ _ _ _ _ w452 _ _ _ _ _ _] -> [_ _ _ _ _ _ _ _ w462 _ _ _ _]
          seq-local: [_ _ _ _ _ _ w451 _ _ _ _ _ _] -> [_ _ _ _ _ _ _ _ w461 _ _ _ _]
          seq-local: [_ _ _ _ _ _ _ _ w465 _ _ _ _] -> [_ _ _ _ _ _ _ _ _ _ w476 _ _]
          seq-local: [_ _ _ _ _ _ _ _ w464 _ _ _ _] -> [_ _ _ _ _ _ _ _ _ _ w475 _ _]
          seq-local: [_ _ _ _ _ _ _ _ _ _ w473 _ _] -> [_ _ _ _ _ _ _ _ _ _ _ _ w490]
          seq-local: [_ _ _ _ _ _ _ _ _ _ w472 _ _] -> [_ _ _ _ _ _ _ _ _ _ _ _ w489]
          tunnel: w414 -> [w426 _ _ _ _ _ _ _ _ _ _ _ _]
          tunnel: w413 -> [w419 _ _ _ _ _ _ _ _ _ _ _ _]
          tunnel: w410 -> [w418 _ w432 _ w445 _ w456 _ w466 _ w479 _ _]
          tunnel: [_ _ _ _ _ _ _ _ _ _ _ _ w488] -> w409
          tunnel: [_ _ _ _ _ _ _ _ _ _ _ _ w486] -> w408
          tunnel: w407 -> [_ _ _ _ _ _ _ _ _ _ _ _ w487]
          frame #0 {
            w423 = " PULSe"  # Function Command
            n199 = local read "输出信号波形"() -> (w417:u16)
            n200 = Concatenate Strings(w418, ":FUNC" ("string (\"\")")) -> (w424:string)
            n201 = Pick Line(string ("")=w424, multi-line string=w423, line index=w417) -> (output string=w422:string)
            n202 = VISA Write(VISA resource name=w426, write buffer=w422, error in (no error)=w419) -> (VISA resource name out=w421:refnum<visa-resource-name>, error out=w420:errorcluster)  [unwired: 1 out]
          }
          frame #1 {
            n203 = Wait (ms)(milliseconds to wait=u32 150) -> ()  [unwired: 1 out]
          }
          frame #2 {
            n204 = Number To Fractional String(use system decimal point (T)=TRUE ("使用系统小数点(T)"), number=1.0 ("数字")) -> (F-format string=w430:string)  [unwired: 2 in]
            n205 = Concatenate Strings ("连接字符串")(w432, ":VOLTage：HIGH ", w430) -> (w429:string)
            n206 = VISA Write(VISA resource name=w436, write buffer=w429, error in (no error)=w435) -> (VISA resource name out=w434:refnum<visa-resource-name>, error out=w433:errorcluster)  [unwired: 1 out]
          }
          frame #3 {
            n207 = Wait (ms)(milliseconds to wait=u32 150) -> ()  [unwired: 1 out]
          }
          frame #4 {
            # "1 电压偏置"
            n208 = Number To Fractional String(use system decimal point (T)=TRUE ("使用系统小数点(T)"), number=0.0 ("数字")) -> (F-format string=w443:string)  [unwired: 2 in]
            n209 = Concatenate Strings(w445, ":VOLTage:LOW ", w443) -> (w444:string)
            n210 = VISA Write(VISA resource name=w439, write buffer=w444, error in (no error)=w440) -> (VISA resource name out=w448:refnum<visa-resource-name>, error out=w447:errorcluster)  [unwired: 1 out]
          }
          frame #5 {
            n211 = Wait (ms)(milliseconds to wait=u32 150) -> ()  [unwired: 1 out]
          }
          frame #6 {
            n212 = local read "channel输出口"() -> (w454:i32)
            n213 = Pick Line(multi-line string=":OUTP1:IMPedance \n:OUTP2:IMPedance " ("write buffer"), line index=w454) -> (output string=w453:string)  [unwired: 1 in]
            n214 = Concatenate Strings ("连接字符串")(w456, w453, "INFINITY") -> (w457:string)
            n215 = VISA Write(VISA resource name=w459, write buffer=w457, error in (no error)=w458) -> (VISA resource name out=w452:refnum<visa-resource-name>, error out=w451:errorcluster)  [unwired: 1 out]
          }
          frame #7 {
            n216 = Wait (ms)(milliseconds to wait=u32 150) -> ()  [unwired: 1 out]
          }
          frame #8 {
            n217 = Number To Fractional String(use system decimal point (T)=TRUE ("使用系统小数点(T)"), number=0.0 ("数字")) -> (F-format string=w469:string)  [unwired: 2 in]
            n218 = Concatenate Strings(w466, ":PULSe:DELay ", w469) -> (w467:string)
            n219 = VISA Write(VISA resource name=w462, write buffer=w467, error in (no error)=w461) -> (VISA resource name out=w465:refnum<visa-resource-name>, error out=w464:errorcluster)  [unwired: 1 out]
          }
          frame #9 {
            n220 = Wait (ms)(milliseconds to wait=u32 150) -> ()  [unwired: 1 out]
          }
          frame #10 {
            w480 = ":LEADing\n:TRAiling "  # Channel
            w484 = ":PULSe:TRANsition"  # VOLTage:Offset
            n221 = local read "上升下降沿"() -> (w481:i32)
            n222 = Pick Line(multi-line string=w480, line index=w481) -> (output string=w477:string)  [unwired: 1 in]
            n223 = Number To Fractional String(use system decimal point (T)=TRUE ("使用系统小数点(T)"), number=0.0 ("数字")) -> (F-format string=w478:string)  [unwired: 2 in]
            n224 = Concatenate Strings(w479, w484, w477, w478) -> (w482:string)
            n225 = VISA Write(VISA resource name=w476, write buffer=w482, error in (no error)=w475) -> (VISA resource name out=w473:refnum<visa-resource-name>, error out=w472:errorcluster)  [unwired: 1 out]
          }
          frame #11 {
            n226 = Wait (ms)(milliseconds to wait=u32 150) -> ()  [unwired: 1 out]
          }
          frame #12 {
            n227 = case shown="假" w487 {
              tunnel: w490 -> [w498 w499]
              tunnel: [w497 w506] -> w486
              tunnel: w489 -> [w496 w504]
              tunnel: [w495 w505] -> w488
              frame True {
                n228 = local write "Output"(TRUE ("布尔")) -> ()
                n229 = local read "channel输出口"() -> (w492:i32)
                n230 = Pick Line(multi-line string=":OUTP1 ON\n:OUTP2 ON" ("write buffer"), line index=w492) -> (output string=w491:string)  [unwired: 1 in]
                n231 = VISA Write(VISA resource name=w498, write buffer=w491, error in (no error)=w496) -> (VISA resource name out=w495:refnum<visa-resource-name>, error out=w497:errorcluster)  [unwired: 1 out]
              }
              frame False {
                n232 = local read "channel输出口"() -> (w501:i32)
                n233 = Pick Line(multi-line string=":OUTP1 OFF\n:OUTP2 OFF" ("write buffer"), line index=w501) -> (output string=w500:string)  [unwired: 1 in]
                n234 = VISA Write(VISA resource name=w499, write buffer=w500, error in (no error)=w504) -> (VISA resource name out=w505:refnum<visa-resource-name>, error out=w506:errorcluster)  [unwired: 1 out]
                n235 = local write "Output"(FALSE ("布尔")) -> ()
              }
            }
          }
        }
        n236 = VISA Close(VISA resource name=w409, error in (no error)=w408) -> (error out=→"output control error  4":errorcluster)
      }
    }
    n237 = case shown="真" "设置参数" {
      frame False {
      }
      frame True {
        w513 = " :SOUR1\n :SOUR2"  # Channel
        n238 = local read "VISA 信号发生器"() -> (w515:refnum<visa-resource-name>)
        n239 = local read "channel输出口"() -> (w514:i32)
        n240 = case shown="1" w514 {
          tunnel: [1 0] -> w507
          frame 0, Default {
          }
          frame 1 {
          }
        }
        n241 = VISA Open(VISA resource name=w515) -> (VISA resource name=w518:refnum<visa-resource-name>, error out=w519:errorcluster)  [unwired: 4 in]
        n242 = Pick Line(multi-line string=w513, line index=w507) -> (output string=w508:string)  [unwired: 1 in]
        n243 = Pick Line(multi-line string=w513, line index=w514) -> (output string=w516:string)  [unwired: 1 in]
        n244 = stacked-sequence {
          seq-local: [w615 _ _ _ _ _ _ _ _ _ _ _ _ _ _] -> [_ _ w630 _ _ _ _ _ _ _ _ _ _ _ _]
          seq-local: [w614 _ _ _ _ _ _ _ _ _ _ _ _ _ _] -> [_ _ w629 _ _ _ _ _ _ _ w668 _ _ _ _]
          seq-local: [_ _ w628 _ _ _ _ _ _ _ _ _ _ _ _] -> [_ _ _ _ w639 _ _ _ _ _ _ _ _ _ _]
          seq-local: [_ _ w627 _ _ _ _ _ _ _ _ _ _ _ _] -> [_ _ _ _ w638 _ _ _ _ _ _ _ _ _ _]
          seq-local: [_ _ _ _ w637 _ _ _ _ _ _ _ _ _ _] -> [_ _ _ _ _ _ w645 _ _ _ _ _ _ _ _]
          seq-local: [_ _ _ _ w634 _ _ _ _ _ _ _ _ _ _] -> [_ _ _ _ _ _ w644 _ _ _ _ _ _ _ _]
          seq-local: [_ _ _ _ _ _ w652 _ _ _ _ _ _ _ _] -> [_ _ _ _ _ _ _ _ w663 _ _ _ _ _ _]
          seq-local: [_ _ _ _ _ _ w651 _ _ _ _ _ _ _ _] -> [_ _ _ _ _ _ _ _ w662 _ _ _ _ _ _]
          seq-local: [_ _ _ _ _ _ _ _ w656 _ _ _ _ _ _] -> [_ _ _ _ _ _ _ _ _ _ w669 _ _ _ _]
          seq-local: [_ _ _ _ _ _ _ _ w655 _ _ _ _ _ _] -> [_ _ _ _ _ _ _ _ _ _ _ _ _ _ _]
          seq-local: [_ _ _ _ _ _ _ _ _ _ w665 _ _ _ _] -> [_ _ _ _ _ _ _ _ _ _ _ _ w679 _ _]
          seq-local: [_ _ _ _ _ _ _ _ _ _ w666 _ _ _ _] -> [_ _ _ _ _ _ _ _ _ _ _ _ w678 _ _]
          seq-local: [_ _ _ _ _ _ _ _ _ _ _ _ w677 _ _] -> [_ _ _ _ _ _ _ _ _ _ _ _ _ _ w690]
          seq-local: [_ _ _ _ _ _ _ _ _ _ _ _ w676 _ _] -> [_ _ _ _ _ _ _ _ _ _ _ _ _ _ w689]
          tunnel: w518 -> [w620 _ _ _ _ _ _ _ _ _ _ _ _ _ _]
          tunnel: w519 -> [w613 _ _ _ _ _ _ _ _ _ _ _ _ _ _]
          tunnel: w516 -> [w612 _ w626 _ w633 _ w649 _ w660 _ w670 _ w680 _ w693]
          tunnel: [_ _ _ _ _ _ _ _ _ _ _ _ _ _ w688] -> w512
          tunnel: [_ _ _ _ _ _ _ _ _ _ _ _ _ _ w687] -> w511
          frame #0 {
            w617 = " PULSe"  # Function Command
            n245 = local read "输出信号波形"() -> (w611:u16)
            n246 = Concatenate Strings(w612, ":FUNC" ("string (\"\")")) -> (w618:string)
            n247 = Pick Line(string ("")=w618, multi-line string=w617, line index=w611) -> (output string=w616:string)
            n248 = VISA Write(VISA resource name=w620, write buffer=w616, error in (no error)=w613) -> (VISA resource name out=w615:refnum<visa-resource-name>, error out=w614:errorcluster)  [unwired: 1 out]
          }
          frame #1 {
            n249 = Wait (ms)(milliseconds to wait=u32 150) -> ()  [unwired: 1 out]
          }
          frame #2 {
            n250 = Number To Fractional String(use system decimal point (T)=TRUE ("使用系统小数点(T)"), number="低电平/V") -> (F-format string=w624:string)  [unwired: 2 in]
            n251 = Concatenate Strings ("连接字符串")(w626, ":VOLTage:LOW ", w624) -> (w623:string)
            n252 = VISA Write(VISA resource name=w630, write buffer=w623, error in (no error)=w629) -> (VISA resource name out=w628:refnum<visa-resource-name>, error out=w627:errorcluster)  [unwired: 1 out]
          }
          frame #3 {
            n253 = Wait (ms)(milliseconds to wait=u32 150) -> ()  [unwired: 1 out]
          }
          frame #4 {
            # "1 频率"
            n254 = Concatenate Strings(w633, ":FREQ ") -> (w640:string)
            n255 = Format Into String ("格式化写入字符串")(initial string=w640, "频率/Hz") -> (resulting string=w641:string)  [unwired: 2 in, 1 out]
            n256 = VISA Write(VISA resource name=w639, write buffer=w641, error in (no error)=w638) -> (VISA resource name out=w637:refnum<visa-resource-name>, error out=w634:errorcluster)  [unwired: 1 out]
          }
          frame #5 {
            n257 = Wait (ms)(milliseconds to wait=u32 150) -> ()  [unwired: 1 out]
          }
          frame #6 {
            n258 = Number To Fractional String(use system decimal point (T)=TRUE ("使用系统小数点(T)"), number="高电平/V") -> (F-format string=w646:string)  [unwired: 2 in]
            n259 = Concatenate Strings(w649, ":VOLTage:HIGH ", w646) -> (w648:string)
            n260 = VISA Write(VISA resource name=w645, write buffer=w648, error in (no error)=w644) -> (VISA resource name out=w652:refnum<visa-resource-name>, error out=w651:errorcluster)  [unwired: 1 out]
          }
          frame #7 {
            n261 = Wait (ms)(milliseconds to wait=u32 150) -> ()  [unwired: 1 out]
          }
          frame #8 {
            n262 = local read "channel输出口"() -> (w658:i32)
            n263 = Pick Line(multi-line string=":OUTP1:IMPedance \n:OUTP2:IMPedance " ("write buffer"), line index=w658) -> (output string=w657:string)  [unwired: 1 in]
            n264 = Concatenate Strings ("连接字符串")(w660, w657, "INFINITY") -> (w661:string)
            n265 = VISA Write(VISA resource name=w663, write buffer=w661, error in (no error)=w662) -> (VISA resource name out=w656:refnum<visa-resource-name>, error out=w655:errorcluster)  [unwired: 1 out]
          }
          frame #9 {
            n266 = Wait (ms)(milliseconds to wait=u32 150) -> ()  [unwired: 1 out]
          }
          frame #10 {
            n267 = Number To Fractional String(use system decimal point (T)=TRUE ("使用系统小数点(T)"), number="占空比/%") -> (F-format string=w672:string)  [unwired: 2 in]
            n268 = Concatenate Strings(w670, ":PULSe:DCYCle ", w672) -> (w667:string)
            n269 = VISA Write(VISA resource name=w669, write buffer=w667, error in (no error)=w668) -> (VISA resource name out=w665:refnum<visa-resource-name>, error out=w666:errorcluster)  [unwired: 1 out]
          }
          frame #11 {
            n270 = Wait (ms)(milliseconds to wait=u32 150) -> ()  [unwired: 1 out]
          }
          frame #12 {
            n271 = Number To Fractional String(use system decimal point (T)=TRUE ("使用系统小数点(T)"), number="延时/s") -> (F-format string=w683:string)  [unwired: 2 in]
            n272 = Concatenate Strings(w680, ":PULSe:DELay ", w683) -> (w681:string)
            n273 = VISA Write(VISA resource name=w679, write buffer=w681, error in (no error)=w678) -> (VISA resource name out=w677:refnum<visa-resource-name>, error out=w676:errorcluster)  [unwired: 1 out]
          }
          frame #13 {
            n274 = Wait (ms)(milliseconds to wait=u32 150) -> ()  [unwired: 1 out]
          }
          frame #14 {
            w694 = ":LEADing\n:TRAiling "  # Channel
            w699 = ":PULSe:TRANsition"  # VOLTage:Offset
            n275 = local read "上升下降沿"() -> (w695:i32)
            n276 = Pick Line(multi-line string=w694, line index=w695) -> (output string=w691:string)  [unwired: 1 in]
            n277 = Number To Fractional String(use system decimal point (T)=TRUE ("使用系统小数点(T)"), number="上升下降沿/s") -> (F-format string=w692:string)  [unwired: 2 in]
            n278 = Concatenate Strings(w693, w699, w691, w692) -> (w696:string)
            n279 = VISA Write(VISA resource name=w690, write buffer=w696, error in (no error)=w689) -> (VISA resource name out=w688:refnum<visa-resource-name>, error out=w687:errorcluster)  [unwired: 1 out]
          }
        }
        n280 = stacked-sequence {
          seq-local: [w526 _ _ _ _ _ _ _ _ _ _ _ _ _ _] -> [_ _ w541 _ _ _ _ _ _ _ _ _ _ _ _]
          seq-local: [w525 _ _ _ _ _ _ _ _ _ _ _ _ _ _] -> [_ _ w540 _ _ _ _ _ _ _ w579 _ _ _ _]
          seq-local: [_ _ w539 _ _ _ _ _ _ _ _ _ _ _ _] -> [_ _ _ _ w550 _ _ _ _ _ _ _ _ _ _]
          seq-local: [_ _ w538 _ _ _ _ _ _ _ _ _ _ _ _] -> [_ _ _ _ w549 _ _ _ _ _ _ _ _ _ _]
          seq-local: [_ _ _ _ w548 _ _ _ _ _ _ _ _ _ _] -> [_ _ _ _ _ _ w556 _ _ _ _ _ _ _ _]
          seq-local: [_ _ _ _ w545 _ _ _ _ _ _ _ _ _ _] -> [_ _ _ _ _ _ w555 _ _ _ _ _ _ _ _]
          seq-local: [_ _ _ _ _ _ w563 _ _ _ _ _ _ _ _] -> [_ _ _ _ _ _ _ _ w574 _ _ _ _ _ _]
          seq-local: [_ _ _ _ _ _ w562 _ _ _ _ _ _ _ _] -> [_ _ _ _ _ _ _ _ w573 _ _ _ _ _ _]
          seq-local: [_ _ _ _ _ _ _ _ w568 _ _ _ _ _ _] -> [_ _ _ _ _ _ _ _ _ _ w580 _ _ _ _]
          seq-local: [_ _ _ _ _ _ _ _ w567 _ _ _ _ _ _] -> [_ _ _ _ _ _ _ _ _ _ _ _ _ _ _]
          seq-local: [_ _ _ _ _ _ _ _ _ _ w576 _ _ _ _] -> [_ _ _ _ _ _ _ _ _ _ _ _ w590 _ _]
          seq-local: [_ _ _ _ _ _ _ _ _ _ w577 _ _ _ _] -> [_ _ _ _ _ _ _ _ _ _ _ _ w589 _ _]
          seq-local: [_ _ _ _ _ _ _ _ _ _ _ _ w588 _ _] -> [_ _ _ _ _ _ _ _ _ _ _ _ _ _ w603]
          seq-local: [_ _ _ _ _ _ _ _ _ _ _ _ w587 _ _] -> [_ _ _ _ _ _ _ _ _ _ _ _ _ _ w602]
          tunnel: w512 -> [w531 _ _ _ _ _ _ _ _ _ _ _ _ _ _]
          tunnel: w511 -> [w524 _ _ _ _ _ _ _ _ _ _ _ _ _ _]
          tunnel: w508 -> [w523 _ w537 _ w544 _ w560 _ w571 _ w581 _ w591 _ w598]
          tunnel: [_ _ _ _ _ _ _ _ _ _ _ _ _ _ w601] -> w510
          tunnel: [_ _ _ _ _ _ _ _ _ _ _ _ _ _ w600] -> w509
          tunnel: w507 -> [_ _ _ _ _ _ _ _ w565 _ _ _ _ _ _]
          frame #0 {
            w528 = " PULSe"  # Function Command
            n281 = Concatenate Strings(w523, ":FUNC" ("string (\"\")")) -> (w529:string)
            n282 = Pick Line(string ("")=w529, multi-line string=w528, line index="输出信号波形 2") -> (output string=w527:string)
            n283 = VISA Write(VISA resource name=w531, write buffer=w527, error in (no error)=w524) -> (VISA resource name out=w526:refnum<visa-resource-name>, error out=w525:errorcluster)  [unwired: 1 out]
          }
          frame #1 {
            n284 = Wait (ms)(milliseconds to wait=u32 150) -> ()  [unwired: 1 out]
          }
          frame #2 {
            n285 = Number To Fractional String(use system decimal point (T)=TRUE ("使用系统小数点(T)"), number="低电平/V 2") -> (F-format string=w535:string)  [unwired: 2 in]
            n286 = Concatenate Strings ("连接字符串")(w537, ":VOLTage:LOW ", w535) -> (w534:string)
            n287 = VISA Write(VISA resource name=w541, write buffer=w534, error in (no error)=w540) -> (VISA resource name out=w539:refnum<visa-resource-name>, error out=w538:errorcluster)  [unwired: 1 out]
          }
          frame #3 {
            n288 = Wait (ms)(milliseconds to wait=u32 150) -> ()  [unwired: 1 out]
          }
          frame #4 {
            # "1 频率"
            n289 = Concatenate Strings(w544, ":FREQ ") -> (w551:string)
            n290 = Format Into String ("格式化写入字符串")(initial string=w551, "频率/Hz 2") -> (resulting string=w552:string)  [unwired: 2 in, 1 out]
            n291 = VISA Write(VISA resource name=w550, write buffer=w552, error in (no error)=w549) -> (VISA resource name out=w548:refnum<visa-resource-name>, error out=w545:errorcluster)  [unwired: 1 out]
          }
          frame #5 {
            n292 = Wait (ms)(milliseconds to wait=u32 150) -> ()  [unwired: 1 out]
          }
          frame #6 {
            n293 = Number To Fractional String(use system decimal point (T)=TRUE ("使用系统小数点(T)"), number="高电平/V 2") -> (F-format string=w557:string)  [unwired: 2 in]
            n294 = Concatenate Strings(w560, ":VOLTage:HIGH ", w557) -> (w559:string)
            n295 = VISA Write(VISA resource name=w556, write buffer=w559, error in (no error)=w555) -> (VISA resource name out=w563:refnum<visa-resource-name>, error out=w562:errorcluster)  [unwired: 1 out]
          }
          frame #7 {
            n296 = Wait (ms)(milliseconds to wait=u32 150) -> ()  [unwired: 1 out]
          }
          frame #8 {
            n297 = Pick Line(multi-line string=":OUTP1:IMPedance \n:OUTP2:IMPedance " ("write buffer"), line index=w565) -> (output string=w569:string)  [unwired: 1 in]
            n298 = Concatenate Strings ("连接字符串")(w571, w569, "INFINITY") -> (w572:string)
            n299 = VISA Write(VISA resource name=w574, write buffer=w572, error in (no error)=w573) -> (VISA resource name out=w568:refnum<visa-resource-name>, error out=w567:errorcluster)  [unwired: 1 out]
          }
          frame #9 {
            n300 = Wait (ms)(milliseconds to wait=u32 150) -> ()  [unwired: 1 out]
          }
          frame #10 {
            n301 = Number To Fractional String(use system decimal point (T)=TRUE ("使用系统小数点(T)"), number="占空比/% 2") -> (F-format string=w583:string)  [unwired: 2 in]
            n302 = Concatenate Strings(w581, ":PULSe:DCYCle ", w583) -> (w578:string)
            n303 = VISA Write(VISA resource name=w580, write buffer=w578, error in (no error)=w579) -> (VISA resource name out=w576:refnum<visa-resource-name>, error out=w577:errorcluster)  [unwired: 1 out]
          }
          frame #11 {
            n304 = Wait (ms)(milliseconds to wait=u32 150) -> ()  [unwired: 1 out]
          }
          frame #12 {
            n305 = Number To Fractional String(use system decimal point (T)=TRUE ("使用系统小数点(T)"), number="延时/s 2") -> (F-format string=w594:string)  [unwired: 2 in]
            n306 = Concatenate Strings(w591, ":PULSe:DELay ", w594) -> (w592:string)
            n307 = VISA Write(VISA resource name=w590, write buffer=w592, error in (no error)=w589) -> (VISA resource name out=w588:refnum<visa-resource-name>, error out=w587:errorcluster)  [unwired: 1 out]
          }
          frame #13 {
            n308 = Wait (ms)(milliseconds to wait=u32 150) -> ()  [unwired: 1 out]
          }
          frame #14 {
            w606 = ":LEADing\n:TRAiling "  # Channel
            w610 = ":PULSe:TRANsition"  # VOLTage:Offset
            n309 = Pick Line(multi-line string=w606, line index="上升下降沿 2") -> (output string=w604:string)  [unwired: 1 in]
            n310 = Number To Fractional String(use system decimal point (T)=TRUE ("使用系统小数点(T)"), number="上升下降沿/s 2") -> (F-format string=w605:string)  [unwired: 2 in]
            n311 = Concatenate Strings(w598, w610, w604, w605) -> (w607:string)
            n312 = VISA Write(VISA resource name=w603, write buffer=w607, error in (no error)=w602) -> (VISA resource name out=w601:refnum<visa-resource-name>, error out=w600:errorcluster)  [unwired: 1 out]
          }
        }
        n313 = VISA Close(VISA resource name=w510, error in (no error)=w509) -> (error out=→"configure error out":errorcluster)
      }
    }
    n314 = event shown="[1] \"照明光\": 值改变" {
      selector: _ -> [_ _]
      dyn-events: _ -> [_ _]
      timeout: 0 -> [_ _]
      tunnel: "照明光" -> [_ w60]
      event Timeout {
        n315 = event-data() -> ()  [unwired: 1 in, 3 out]
      }
      event "照明光": Value Change {
        n316 = event-data() -> ()  [unwired: 1 in, 6 out]
        n317 = local read "stop bits (10: 1 bit)"() -> (w73:u16)
        n318 = local read "parity (0:none)"() -> (w72:enum16{"None", "Odd", "Even", "Mark", "Space"})
        n319 = local read "照明光VISA"() -> (w69:refnum<visa-resource-name>)
        n320 = local read "baud rate"() -> (w70:u32)
        n321 = local read "data bits (8)"() -> (w71:u16)
        n322 = call-poly "VISA Configure Serial Port"("VISA resource name"=w69, "baud rate (9600)"=w70, "data bits (8)"=w71, "parity (0:none)"=w72, "stop bits (10: 1 bit)"=w73) -> ("VISA resource name out"=w66:refnum<visa-resource-name>, "error out"=w65:errorcluster)  [unwired: 9 in]
        n323 = call <vilib>:"Simple Error Handler.vi"("error in (no error)"=w65) -> ()  [unwired: 4 in, 5 out]
        n324 = VISA Open(access mode=0, error in (no error)=w65, VISA resource name=w66) -> (VISA resource name=w68:refnum<visa-resource-name>, error out=w67:errorcluster)  [unwired: 2 in]
        n325 = stacked-sequence {
          tunnel: w68 -> [w78]
          tunnel: w67 -> [w77]
          tunnel: [w76] -> w63
          tunnel: [w75] -> w64
          tunnel: w60 -> [w74]
          frame #0 {
            n326 = case shown="假" w74 {
              tunnel: w78 -> [w84 w94]
              tunnel: [w82 w93] -> w76
              tunnel: w77 -> [w83 w92]
              tunnel: [w81 w91] -> w75
              frame False {
                n327 = Concatenate Strings(" \u0001\u0001¢", "\r") -> (w85:string)
                n328 = VISA Write(VISA resource name=w84, write buffer=w85, error in (no error)=w83) -> (VISA resource name out=w82:refnum<visa-resource-name>, error out=w81:errorcluster)  [unwired: 1 out]
                n329 = Wait (ms)(milliseconds to wait=50) -> ()  [unwired: 1 out]
              }
              frame True {
                w87 = " \u0001\u0000¡"  # Channel
                n330 = Wait (ms)(milliseconds to wait=50) -> ()  [unwired: 1 out]
                n331 = Concatenate Strings(w87, "\r") -> (w88:string)
                n332 = VISA Write(VISA resource name=w94, write buffer=w88, error in (no error)=w92) -> (VISA resource name out=w93:refnum<visa-resource-name>, error out=w91:errorcluster)  [unwired: 1 out]
              }
            }
          }
        }
        n333 = VISA Close(VISA resource name=w63, error in (no error)=w64) -> (error out=w62:errorcluster)
        n334 = call <vilib>:"Simple Error Handler.vi"("error in (no error)"=w62) -> ()  [unwired: 4 in, 5 out]
      }
    }
  }
  n335 = flat-sequence {
    frame #0 {
      "Backlight" <- i32[][] [] ("Backlight")
    }
    frame #1 {
      w701 = FALSE
      # "删除背景光控件\n初始值设定"
      n336 = local write "cut backlight"(w701) -> ()
      "backlight" <- w701
    }
  }
  n337 = stacked-sequence {
    seq-local: [_ _ _ w722 _ _ _ _] -> [_ _ _ _ w740 w760 w763 w965]
    seq-local: [_ _ _ w721 _ _ _ _] -> [_ _ _ _ w741 w761 w762 w966]
    frame #0 {
      # "initialize all variables"
      n338 = property on="initialize" class="Bool"("Désactivé"=u8 0) -> ()  [unwired: 2 in, 2 out]
      n339 = property on="Acquire" class="Bool"("Visible"=FALSE) -> ()  [unwired: 2 in, 2 out]
      n340 = property on="Setup" class="Bool"("Visible"=FALSE) -> ()  [unwired: 2 in, 2 out]
      n341 = local write "indicator"("" ("indicator")) -> ()
      n342 = local write "initialized ?"(FALSE ("initialized ?")) -> ()
      n343 = local write "Continuous"(FALSE ("Continuous")) -> ()
      n344 = local write "Close"(FALSE ("Close")) -> ()
      n345 = property on="Device Name" class="Ring (严格)"("Désactivé"=u8 0) -> ()  [unwired: 2 in, 2 out]
      n346 = property on="Continuous" class="Bool (严格)"("Visible"=FALSE) -> ()  [unwired: 2 in, 2 out]
      n347 = local write "Commande tab"(T1."Settings" ("Commande tab")) -> ()
    }
    frame #1 {
      # "Read Uniq ID"
      n348 = stacked-sequence {
        frame #0 {
          n349 = call "read detector uniq-id.vi"() -> ("nbr of components"=w714:i32, "UniqueID"=w713:string[], "Name"=w712:string[])  [unwired: 4 out]
          n350 = for {
            N: w714 -> [_]
            tunnel: w713 -> [w716]
            tunnel: w712 -> [w715]
            n351 = property on="Device Name" class="Ring (严格)"("Chaînes []"=w715) -> ()  [unwired: 2 in, 2 out]
            n352 = property on="Uniques ID" class="Ring (严格)"("Chaînes []"=w716) -> ()  [unwired: 2 in, 2 out]
          }
        }
      }
    }
    frame #2 {
      n353 = while {
        stop <- "initialize" stop-if-true
        n354 = local read "Device Name"() -> (w719:u16)
        n355 = local write "Uniques ID"(w719) -> ()
        n356 = local read "Close"() -> (w717:bool)
        n357 = Stop(stop? (T)=w717) -> ()
        n358 = Wait Until Next ms Multiple(millisecond multiple=u32 100 ("n millisecondes")) -> ()  [unwired: 1 out]
      }
    }
    frame #3 {
      n359 = stacked-sequence {
        tunnel: [_ w729 _ _] -> w722
        tunnel: [_ w728 _ _] -> w721
        frame #0 {
          n360 = local write "indicator"("Initializing ..." ("indicator")) -> ()
        }
        frame #1 {
          n361 = local read "Uniques ID"() -> (w726:u16)
          n362 = property on="Uniques ID" class="Ring (严格)"() -> ("Chaînes []"=w727:string[])  [unwired: 2 in, 2 out]
          n363 = Index Array(array=w727, index=w726) -> (element=w725:string)
          n364 = call "Initialize CCD.vi"("Unique id:"=w725) -> ("activeYPixels"=→"Y Pixels:":i32, "JYCCDLib.IJYCCDReqd"=w728:refnum<k7>, "activeXPixels"=→"X Pixels:":i32, "sortie d'erreur"=w729:errorcluster, "FirmwareVersion"=→"Firmware\nVersion":string)  [unwired: 3 out]
        }
        frame #2 {
          n365 = property on="initialize" class="Bool"("Désactivé"=u8 2) -> ()  [unwired: 2 in, 2 out]
          n366 = property on="Device Name" class="Ring (严格)"("Désactivé"=u8 2) -> ()  [unwired: 2 in, 2 out]
          n367 = local write "Continuous"(FALSE ("Continuous")) -> ()
          n368 = property on="Setup" class="Bool"("Visible"=TRUE) -> ()  [unwired: 2 in, 2 out]
        }
        frame #3 {
          n369 = local write "initialized ?"(TRUE ("initialized ?")) -> ()
          n370 = local write "indicator"("Initialized !" ("indicator")) -> ()
        }
      }
    }
    frame #4 {
      # "Actually not working"
      # "Read ADC and GAIN"
      n371 = case shown="真" "Constante de condition\n(Voir l'aide contextuelle)" {
        tunnel: w741 -> [_ w751]
        tunnel: w740 -> [_ w750]
        frame False {
        }
        frame True {
          # "Read Input supported trigger"
          n372 = call "Trigger - Get Supported Input.vi"("JYCCDLib.IJYCCDReqd"=w751, "Error Input"=w750) -> ("trigAddress"=w745:i32, "eventPtr"=w746:i32, "trigEventString"=w749:string, "trigSigType"=w748:i32, "trigSigTypeString"=w747:string)  [unwired: 4 out]
          n373 = local write "trigSigTypeString"(w747) -> ()
          n374 = local write "trigAddress"(w745) -> ()
          n375 = local write "Trigger Type :"(w746) -> ()
          n376 = local write "trigEventString"(w749) -> ()
          n377 = local write "Signal type :"(w748) -> ()
        }
      }
      n378 = call "Init ADC & Gain.vi"("JYCCDLib.IJYCCDReqd"=w741, "input error"=w740) -> ("ADC Number"=w739:i32[], "ADC description"=w744:string[], "Gain Number"=w742:i32[], "Gain description"=w743:string[])
      n379 = local write "Gain Number"(w742) -> ()
      n380 = local write "ADC Number"(w739) -> ()
      n381 = stacked-sequence {
        tunnel: w744 -> [w752 _]
        tunnel: w743 -> [_ w753]
        frame #0 {
          n382 = property on="ADC" class="Ring (严格)"("Chaînes []"=w752) -> ()  [unwired: 2 in, 2 out]
        }
        frame #1 {
          n383 = property on="GAIN" class="Ring (严格)"("Chaînes []"=w753) -> ()  [unwired: 2 in, 2 out]
        }
      }
    }
    frame #5 {
      # "IS multi Accumulation Supported ?"
      n384 = call "MultiAccu - Is Supported.vi"("Error In"=w760, "JYCCDLib.IJYCCDReqd"=w761) -> ("IsOperatingModeSupported"=w754:bool)  [unwired: 3 out]
      n385 = Select(t=0, s=w754, f=2) -> (s? t:f=w757:i32)
      n386 = Select(t=FALSE, s=w754, f=w754) -> (s? t:f=w756:bool)
      n387 = local write "Multi Accumulation mode:"(w756) -> ()
      n388 = property on="Multi Accumulation mode:" class="Bool (严格)"("Désactivé"=w757) -> ()  [unwired: 2 in, 2 out]
      n389 = property on="Multi Accumulation mode:" class="Bool (严格)"("Désactivé"=w757) -> ()  [unwired: 2 in, 2 out]
    }
    frame #6 {
      n390 = while {
        tunnel: w762 -> [w770]
        tunnel: w763 -> [w769]
        stop <- "Close" stop-if-true
        n391 = local read "Continuous"() -> (w771:bool)
        n392 = case shown="假" "Reformat" {
          frame False {
          }
          frame True {
            n393 = local read "Y Pixels:"() -> (w943:i32)
            n394 = local read "X Pixels:"() -> (w945:i32)
            n395 = call "Spectral Reformat CCD area.vi"("Y Pixels:"=w943, "X Pixels:"=w945, "numAreas"="Number of Areas :") -> ("areas :"=→"areas :":i32[][])  [unwired: 3 out]
          }
        }
        n396 = local read "Accumulations:"() -> (w766:u16)
        n397 = Or(x="Acquire", y=w771) -> (x .or. y?=w768:bool)
        n398 = case shown="真" w768 {
          tunnel: w770 -> [_ w783]
          tunnel: w769 -> [_ w782]
          tunnel: "Enable InputTriggers :" -> [_ w781]
          tunnel: "Multi Accumulation mode:" -> [_ w780]
          tunnel: w766 -> [_ w779]
          tunnel: "MultiAcqShutterMode" -> [_ w778]
          frame False {
          }
          frame True {
            n399 = stacked-sequence {
              seq-local: [_ _ w796 _ _] -> [_ _ _ w869 _]
              seq-local: [_ _ _ w842 _] -> [_ _ _ _ w909]
              tunnel: w783 -> [_ w785 w800 w868 _]
              tunnel: w782 -> [_ w786 w799 w867 _]
              tunnel: w781 -> [_ w787 _ _ _]
              tunnel: w780 -> [_ _ w798 _ _]
              tunnel: w779 -> [_ _ w797 _ _]
              tunnel: w778 -> [_ _ w795 _ _]
              frame #0 {
                n400 = local write "CCD Busy"(TRUE ("CCD Busy")) -> ()
              }
              frame #1 {
                n401 = case shown="真" w787 {
                  tunnel: w786 -> [w788 w794]
                  tunnel: w785 -> [w789 w793]
                  frame False {
                    n402 = call "Trigger - Disable.vi"("Error In"=w788, "JYCCDLib.IJYCCDReqd"=w789) -> ()  [unwired: 6 out]
                  }
                  frame True {
                    n403 = local read "Trigger Type :"() -> (w790:u16)
                    n404 = local read "Signal type :"() -> (w791:enum16{"TTL Rising Edge", "TTL Falling Edge"})
                    n405 = local read "trigAddress"() -> (w792:i32)
                    n406 = call "Trigger - Enable.vi"("Error In"=w794, "sigType"=w791, "event"=w790, "trigAddress"=w792, "JYCCDLib.IJYCCDReqd"=w793) -> ()  [unwired: 3 out]
                  }
                }
              }
              frame #2 {
                n407 = case shown="真" w798 {
                  selector: w798 -> [_ w829]
                  tunnel: w800 -> [w826 w832]
                  tunnel: w799 -> [w825 w831]
                  tunnel: w797 -> [_ w830]
                  tunnel: [u16 1 ("Accumulations:") w830] -> w796
                  tunnel: w795 -> [_ w828]
                  frame False {
                    n408 = call "MultiAccu - Disable.vi"("Error In"=w825, "JYCCDLib.IJYCCDReqd"=w826) -> ()  [unwired: 4 out]
                  }
                  frame True {
                    n409 = call "MultiAccu - Configure.vi"("JYCCDLib.IJYCCDReqd"=w832, "Cleans Before"="Number of Cleans", "Accumulations:"=w830, "MultiAcqHardwareMode"=w829, "MultiAcqShutterMode"=w828, "Error In"=w831) -> ()  [unwired: 1 in, 9 out]
                  }
                }
                n410 = flat-sequence {
                  frame #0 {
                    n411 = Current VI's Path() -> (path=w806:path)
                    n412 = Get Date/Time In Seconds() -> (seconds since 1Jan1904=w808:timestamp)
                    n413 = Strip Path(path=w806) -> (stripped path=w807:path)  [unwired: 1 out]
                    n414 = Path To String(path=w807) -> (string=w809:string)
                    n415 = Format Date/Time String(time format string (%c)="%m.%d" ("时间格式字符串(%c)"), seconds (now)=w808) -> (date/time string=w815:string)  [unwired: 1 in]
                    n416 = Concatenate Strings(w809, "\\Save\\" ("字符串"), w815) -> (w810:string)
                    n417 = String To Path(string=w810) -> (path=w811:path)
                    n418 = call <vilib>:"Check if File or Folder Exists.vi"("path"=w811) -> ("file or folder exists?"=w812:bool, "dup path"=w814:path)  [unwired: 8 in, 1 out]
                    n419 = case shown="真" w812 {
                      tunnel: [w822 w823] -> w813
                      tunnel: w814 -> [w821 w823]
                      tunnel: w815 -> [w820 _]
                      frame False {
                        n420 = Create Folder(prompt (Create Folder)=w820, path (use dialog)=w821) -> (created path=w822:path)  [unwired: 1 in, 2 out]
                      }
                      frame True {
                      }
                    }
                    n421 = Format Date/Time String(time format string (%c)="%y%m%d%H%M%S " ("时间格式字符串(%c)"), seconds (now)=w808) -> (date/time string=w818:string)  [unwired: 1 in]
                    n422 = Path To String(path=w813) -> (string=w816:string)
                    n423 = Concatenate Strings(w816, "\\" ("字符串")) -> (w817:string)
                    n424 = Concatenate Strings(w817, w818) -> (w805:string)
                    n425 = String To Path(string=w805) -> (path=→"最终存储路径 2":path)
                  }
                }
              }
              frame #3 {
                n426 = local read "cut backlight"() -> (w856:bool)
                n427 = local read "backlight"() -> (w855:bool)
                n428 = call "MultiAccu - Acquire spectral.vi"("error in"=w867, "Accumulations:"=w869, "ShutterOpen"="ShutterOpen", "JYCCDLib.IJYCCDReqd"=w868) -> ("Acq Time(ms)"=→"Acq Time(ms)":u32, "Array Out"=w866:i32[][][])  [unwired: 1 out]
                n429 = And(x=w856, y=w855) -> (x .and. y?=w857:bool)
                n430 = call "Array reset dimension.vi"("Area Number"="Area Number to Display", "Array In"=w866) -> ("Array Out"=w858:i32[][])
                n431 = case shown="真" w857 {
                  tunnel: [w905 w906] -> w859
                  tunnel: w858 -> [w905 w907]
                  frame False {
                  }
                  frame True {
                    n432 = local read "Backlight"() -> (w908:i32[][])
                    n433 = Subtract(x=w907, y=w908) -> (x-y=w906:i32[][])
                  }
                }
                n434 = local read "波长范围"() -> (w834:dbl[])
                n435 = local write "Data"(w858) -> ()
                n436 = Index Array(array=w859, index (row)=0 ("禁用的索引 (列)")) -> (element=w860:i32[])  [unwired: 1 in]
                n437 = Reverse 1D Array(array=w860) -> (reversed array=w843:i32[])
                n438 = call "转换至动态数据2"("Array"=w834) -> ("Dynamic Data Type"=w862:dynamicdata)  [unwired: 3 in]
                n439 = call "转换至动态数据"("Array"=w843) -> ("Dynamic Data Type"=w863:dynamicdata)  [unwired: 3 in]
                n440 = call <vilib>:"Median Filter.vi"("left rank"=6, "X"=w843) -> ("Filtered X"=w848:dbl[])  [unwired: 8 in, 1 out]
                n441 = call "Build XY Graph2"("Y Input"=w863, "X Input"=w862) -> ("XY Graph"=w861:cluster{"Y":dbl[], "Y":dbl[]}[])  [unwired: 8 in, 1 out]
                n442 = Subtract(x="拟合终点", y="拟合起点") -> (x-y=w837:i32)
                n443 = local write "Spectrum"(w861) -> ()
                n444 = local read "滤波阈值"() -> (w852:dbl)
                n445 = Array Subset(array=w834, index="拟合起点", length=w837) -> (w840:dbl[])
                n446 = local read "拟合参数"() -> (w833:dbl[])
                n447 = In Range and Coerce(upper limit=w852, x=w848, lower limit=-100.0) -> (In Range?=w851:bool[])  [unwired: 1 out]
                n448 = Not(x=w851) -> (.not. x?=w845:bool[])
                n449 = local read "滤波阈值"() -> (w847:dbl)
                n450 = local write "范围内？"(w851) -> ()
                n451 = local read "X Pixels:"() -> (w849:i32)
                n452 = Or Array Elements(Boolean array=w845) -> (logical OR=w850:bool)
                n453 = case shown="真" w850 {
                  tunnel: w849 -> [_ w892]
                  tunnel: w848 -> [w888 w891]
                  tunnel: [w888 w890] -> w836
                  tunnel: w847 -> [_ w889]
                  frame False {
                  }
                  frame True {
                    n454 = for {
                      N: w892 -> [_]
                      tunnel: w891 -> [w896] mode=indexing
                      tunnel: [w895] -> w890 mode=indexing
                      shift-right: [w895] -> _
                      shift-left: _ -> [w894]
                      tunnel: w889 -> [w893]
                      n455 = Greater?(x=w896, y=w893) -> (0:w898:bool)
                      n456 = Less?(x=w896, y=-100.0) -> (x < y?=w899:bool)
                      n457 = Or(x=w898, y=w899) -> (x .or. y?=w897:bool)
                      n458 = case shown="真" w897 {
                        tunnel: w896 -> [w901 _]
                        tunnel: [w901 w903] -> w895
                        tunnel: w894 -> [_ w904]
                        frame False {
                        }
                        frame True {
                          n459 = call <vilib>:"Median Filter PtByPt.vi"("rank"=5, "x"=w904) -> ("Filtered x"=w903:dbl)  [unwired: 2 in, 1 out]
                        }
                      }
                    }
                  }
                }
                n460 = Array Subset(array=w836, index="拟合起点", length=w837) -> (w839:dbl[])
                n461 = Bundle("波长范围"=w834, "Filtered X"=w836) -> (w835:cluster{"波长范围 ":dbl[], "Filtered X":dbl[]})  [unwired: 1 in]
                n462 = case shown="真" "是否拟合" {
                  tunnel: w839 -> [w872 w878]
                  tunnel: w840 -> [_ w877]
                  tunnel: [w872 w876] -> w854
                  tunnel: w835 -> [_ w874]
                  frame False {
                  }
                  frame True {
                    n463 = call "转换至动态数据7"("Array"=w878) -> ("Dynamic Data Type"=w883:dynamicdata)  [unwired: 3 in]
                    n464 = call "转换至动态数据8"("Array"=w877) -> ("Dynamic Data Type"=w884:dynamicdata)  [unwired: 3 in]
                    n465 = call "曲线拟合2"("Locations"=w884, "Signals"=w883) -> ("best fit"=w881:dynamicdata, "non-linear coefficients"=w882:dynamicdata)  [unwired: 5 in, 3 out]
                    n466 = call "从动态数据转换3"("Dynamic Data Type"=w882) -> ("Array"=w885:dbl[])  [unwired: 3 in]
                    n467 = call "从动态数据转换4"("Dynamic Data Type"=w881) -> ("Array"=w876:dbl[])  [unwired: 3 in]
                    n468 = Index Array(array=w885, index #1=0 ("索引"), index #2=1 ("索引")) -> (element #1=w887:dbl, element #2=w886:dbl)
                    n469 = local write "拟合参数"(w885) -> ()
                    n470 = local write "xc"(w887) -> ()
                    n471 = Bundle(w877, "Array"=w876) -> (w875:cluster{dbl[], "Array":dbl[]})  [unwired: 1 in]
                    n472 = local write "w"(w886) -> ()
                    n473 = Build Array(w874, w875) -> (→"best fit":cluster{"波长范围 ":dbl[], "Array":dbl[]}[])
                  }
                }
                n474 = Build Array(w840, w843, w854, w833) -> (w842:dbl[][])
              }
              frame #4 {
                n475 = case shown="真" "是否保存" {
                  tunnel: w909 -> [_ w913]
                  frame False {
                  }
                  frame True {
                    n476 = Get Date/Time In Seconds() -> (seconds since 1Jan1904=w927:timestamp)
                    n477 = Get Date/Time String(date format (0)=enum16{"short", "long", "abbreviated"}."abbreviated" ("日期格式(0)"), seconds (now)=w927, want seconds? (F)=TRUE ("需要秒？(F)")) -> (date string=w925:string, time string=w926:string)
                    n478 = Search and Replace String(replace all?=TRUE ("替换全部？(F)"), input string=w926, search string=":" ("搜索字符串"), replace string="-" ("替换字符串(\"\")")) -> (result string=w924:string)  [unwired: 4 in, 3 out]
                    n479 = local read "最终存储路径 2"() -> (w928:path)
                    n480 = Path To String(path=w928) -> (string=w931:string)
                    n481 = Concatenate Strings(w931, w925, w924, "光谱" ("字符串"), ".xls" ("字符串")) -> (w930:string)
                    n482 = String To Path(string=w930) -> (path=w929:path)
                    n483 = call-poly <vilib>:"Write Delimited Spreadsheet.vi"("file path (dialog if empty)"=w929, "format (%.3f)"="%.16f", "2D data"=w913, "append to file? (new file:F)"=TRUE ("append to file? (F)"), "transpose? (no:F)"=TRUE ("transpose? (F)")) -> ()  [unwired: 9 in, 2 out]
                  }
                }
                n484 = case shown="真" "Save Backlight" {
                  frame False {
                  }
                  frame True {
                    w932 = TRUE ("删除背景光")
                    n485 = local read "Data"() -> (w934:i32[][])
                    n486 = local write "Backlight"(w934) -> ()
                    n487 = local write "cut backlight"(w932) -> ()
                    n488 = local write "backlight"(w932) -> ()
                    n489 = local write "Save Backlight"(FALSE ("Save Backlight")) -> ()
                  }
                }
                n490 = local write "CCD Busy"(FALSE ("CCD Busy")) -> ()
              }
            }
          }
        }
        n491 = case shown="假" "Setup" {
          tunnel: w769 -> [_ w948]
          tunnel: w770 -> [_ w947]
          frame False {
          }
          frame True {
            n492 = stacked-sequence {
              tunnel: w948 -> [_ w962 _]
              tunnel: w947 -> [_ w950 _]
              frame #0 {
                n493 = local write "indicator"("Setting up the detector" ("indicator")) -> ()
              }
              frame #1 {
                w960 = 1 items=["JYMCD_ACQ_FORMAT_IMAGE", "JYMCD_ACQ_FORMAT_SCAN"] ("Acquisition type")
                n494 = local read "Gain Number"() -> (w955:i32[])
                n495 = local read "GAIN"() -> (w951:u16)
                n496 = local read "ADC Number"() -> (w956:i32[])
                n497 = local read "ADC"() -> (w952:u16)
                n498 = Index Array(array=w955, index=w951) -> (element=w953:i32)
                n499 = Index Array(array=w956, index=w952) -> (element=w954:i32)
                n500 = local read "Number of Areas :"() -> (w958:u16)
                n501 = local read "areas :"() -> (w959:i32[][])
                n502 = call "Setup CCD.vi"("numAreas"=w958, "areas :"=w959, "JYCCDLib.IJYCCDReqd"=w950, "entrée d'erreur (pas d'erreur)"=w962, "Acquisition type"=w960, "Gain"=w953, "Select ADC"=w954, "Integration time(ms)"="Integration time (ms) :") -> ("DataSize"=→"DataSize":i32)  [unwired: 1 out]
                "JYCCDLib.IJYCCDReqd" <- w950
              }
              frame #2 {
                w963 = TRUE ("Visible")
                n503 = property on="Continuous" class="Bool (严格)"("Visible"=w963) -> ()  [unwired: 2 in, 2 out]
                n504 = property on="Acquire" class="Bool"("Visible"=w963) -> ()  [unwired: 2 in, 2 out]
                n505 = local write "indicator"("Ready !" ("indicator")) -> ()
              }
            }
          }
        }
        n506 = case shown="假" "Temperature" {
          tunnel: w770 -> [_ w937]
          tunnel: w769 -> [_ w936]
          frame False {
            n507 = property on="temp graph" class="WFChart (严格)"("Visible"=FALSE) -> ()  [unwired: 2 in, 2 out]
          }
          frame True {
            n508 = stacked-sequence {
              tunnel: w937 -> [_ w942]
              tunnel: w936 -> [_ w941]
              frame #0 {
                n509 = property on="temp graph" class="WFChart (严格)"("Visible"=TRUE) -> ()  [unwired: 2 in, 2 out]
              }
              frame #1 {
                w940 = u16 0 items=["° Celsius", "Kelvin", "° Farenheit"] ("units")
                n510 = call "read temperature.vi"("entrée d'erreur (pas d'erreur)"=w941, "units"=w940, "JYCCDLib.IJYCCDReqd"=w942) -> ("Current Temperature"=w939:dbl)
                n511 = local write "temp graph"(w939) -> ()
              }
            }
          }
        }
        n512 = Wait Until Next ms Multiple(millisecond multiple=u32 50 ("n millisecondes")) -> ()  [unwired: 1 out]
      }
    }
    frame #7 {
      n513 = Close Reference(reference=w966, error in (no error)=w965) -> ()  [unwired: 1 out]
    }
  }
  n514 = stacked-sequence {
    seq-local: [_ _ w976 _ _] -> [_ _ _ w986 w991]
    seq-local: [_ _ w975 _ _] -> [_ _ _ w985 _]
    seq-local: [_ _ _ w984 _] -> [_ _ _ _ _]
    frame #0 {
      n515 = call "Get Monos From Config Browser.vi"() -> ("UniqueIDs"=w971:string[], "Mono ID"=w972:string[])  [unwired: 3 in, 1 out]
      n516 = Build Cluster Array(w972, w971) -> (w969:cluster{"String":string, "String":string}[])
      n517 = property on="Mono ID" class="CmbBox"("Strings And Values []"=w969) -> ()  [unwired: 2 in, 2 out]
      n518 = Index Array(array=w969, index=0) -> (element=w970:cluster{"String":string, "String":string})
      n519 = Unbundle(w970) -> ("String"=w967:string)  [unwired: 1 out]
      "Current UniqueID" <- w967
      n520 = local write "Mono ID"(w967) -> ()
    }
    frame #1 {
      n521 = while {
        stop <- "Connect" stop-if-true
        n522 = local read "Mono ID"() -> (w973:string)
        n523 = local write "Current UniqueID"(w973) -> ()
      }
    }
    frame #2 {
      n524 = local read "Mono ID"() -> (w978:string)
      n525 = call "JYInitMono.vi"("Unique ID"=w978, "Force Init"="Force\nInitialization") -> ("Refnum out"=w976:refnum<k7>, "Initialized"=→"Initialized JY":bool, "error out"=w975:errorcluster)  [unwired: 9 in, 2 out]
    }
    frame #3 {
      n526 = call "Show Current Grating.vi"("Refnum in"=w986, "error in (no error)"=w985) -> ("Gratings"=w987:dbl[], "Grating Index"=w981:i32, "Current Grating"=w983:dbl, "Current Description"=w980:string, "error out"=w984:errorcluster)  [unwired: 5 in, 4 out]
      "Gratings" <- w987
      n527 = local write "Current Grating"(w983) -> ()
      n528 = local write "Current Description"(w980) -> ()
      n529 = Number To Decimal String(number=w987) -> (decimal integer string=w989:string[])  [unwired: 1 in]
      n530 = Number To Decimal String(number=w981) -> (decimal integer string=w982:string)  [unwired: 1 in]
      n531 = property on="Target Grating" class="CmbBox"("Value"=w982) -> ()  [unwired: 2 in, 2 out]
      n532 = Build Cluster Array(w989, string[] ["1", "2", "3"]) -> (w990:cluster{"Numeric":string, string}[])
      n533 = property on="Target Grating" class="CmbBox"("Strings And Values []"=w990) -> ()  [unwired: 2 in, 2 out]
    }
    frame #4 {
      n534 = while {
        tunnel: w991 -> [w993]
        stop <- w992 stop-if-true
        n535 = stacked-sequence {
          seq-local: [w997 _ _ _ _] -> [_ w1004 w1015 _ w1023]
          seq-local: [w996 _ _ _ _] -> [_ w1003 w1014 _ _]
          seq-local: [_ w1002 _ _ _] -> [_ _ _ _ _]
          seq-local: [_ w1001 _ _ _] -> [_ _ _ _ _]
          seq-local: [_ _ w1007 _ _] -> [_ _ _ _ _]
          seq-local: [_ _ w1006 _ _] -> [_ _ _ w1017 _]
          tunnel: w993 -> [w995 _ _ w1018 _]
          frame #0 {
            n536 = call "Show Current Grating.vi"("Refnum in"=w995) -> ("Grating Index"=→"Grating Index":i32, "Current Grating"=→"Current Grating":dbl, "Current Description"=→"Current Description":string, "error out"=w996:errorcluster, "JYMONOLib.IJYMonoReqd"=w997:refnum<k7>)  [unwired: 6 in, 4 out]
          }
          frame #1 {
            n537 = call "JYGetCurrentWL.vi"("error in (no error)"=w1003, "JYMONOLib.IJYMonoReqd"=w1004) -> ("error out"=w1001:errorcluster, "Units"=→"Units":string, "Current WL"=→"Current WL":dbl, "JYMONOLib.IJYMonoReqd 2"=w1002:refnum<k7>)  [unwired: 6 in]
          }
          frame #2 {
            w1012 = u16 1 items=["Entrance", "Exit"] ("Mirror Number")
            w1013 = u16 0 items=["Entrance", "Exit"] ("Mirror Number")
            n538 = call "JYGetMirrorPos.vi"("error in (no error)"=w1014, "Mirror"=w1013, "Refnum In"=w1015) -> ("error out"=w1010:errorcluster, "Current Mirror Position"=→"Entrance Mirror\nPosition":i32, "Refnum Out"=w1011:refnum<k7>)  [unwired: 1 in]
            n539 = call "JYGetMirrorPos.vi"("error in (no error)"=w1010, "Mirror"=w1012, "Refnum In"=w1011) -> ("error out"=w1006:errorcluster, "Current Mirror Position"=→"Exit Mirror\nPosition":i32, "Refnum Out"=w1007:refnum<k7>)  [unwired: 1 in]
          }
          frame #3 {
            w1020 = u16 0 items=["Front Entrance", "Side Entrance", "Front Exit", "Side Exit", "First Intermediate", "Second Intermediate"] ("Slit")
            n540 = call "JYGetSlits.vi"("MonoRefNum IN"=w1018, "Slit"=w1020, "error in (no error)"=w1017) -> ("Units"=→"Units 2":string, "Slit Width"=→"Front Entrance":dbl, "error out"=→"error out":errorcluster)  [unwired: 13 in, 1 out]
          }
          frame #4 {
            n541 = case shown="假" "Move To\nTarget Positions" {
              tunnel: w1023 -> [_ w1024]
              frame False {
              }
              frame True {
                n542 = stacked-sequence {
                  seq-local: [w1026 _ _ _] -> [_ w1032 _ _]
                  seq-local: [_ w1030 _ _] -> [_ _ w1047 _]
                  seq-local: [_ _ w1034 _] -> [_ _ _ w1053]
                  seq-local: [_ _ _ w1050] -> [_ _ _ _]
                  tunnel: w1024 -> [w1028 w1031 w1045 w1054]
                  frame #0 {
                    n543 = property on="Target Grating" class="CmbBox"() -> ("Value"=w1025:string)  [unwired: 2 in, 2 out]
                    n544 = local read "error out"() -> (w1027:errorcluster)
                    n545 = Decimal String To Number(string=w1025) -> (number=w1029:i32)  [unwired: 2 in, 1 out]
                    n546 = call "JYTurret.vi"("error in (no error)"=w1027, "Grating Index"=w1029, "JYMONOLib.IJYMonoReqd"=w1028) -> ("error out"=w1026:errorcluster)  [unwired: 2 out]
                  }
                  frame #1 {
                    # "Move Grating to Target Position"
                    n547 = call "JYMoveToWavelength.vi"("error in (no error)"=w1032, "Target WL"="Target WL", "RefNum In"=w1031) -> ("error out"=w1030:errorcluster)  [unwired: 1 in, 2 out]
                  }
                  frame #2 {
                    w1040 = u16 1 items=["Entrance", "Exit"] ("Mirror Number")
                    w1039 = u16 0 items=["Entrance", "Exit"] ("Mirror Number")
                    w1046 = u16 1 items=["Entrance", "Exit", "Front", "Side"] ("Mirror Number")
                    w1049 = u16 0 items=["Entrance", "Exit", "Front", "Side"] ("Mirror Number")
                    # "Move Mirrors"
                    n548 = call "JYMirrorMove.vi"("error in (no error)"=w1047, "Mirror Position"="Entrance Mirror", "Mirror Number"=w1049, "RefNum In"=w1045) -> ("error out"=w1044:errorcluster)  [unwired: 6 in, 1 out]
                    n549 = call "JYMirrorMove.vi"("error in (no error)"=w1044, "Mirror Position"="Exit Mirror", "Mirror Number"=w1046, "RefNum In"=w1045) -> ("error out"=w1037:errorcluster, "MonoRefNum Out"=w1038:refnum<k7>)  [unwired: 6 in]
                    n550 = call "JYGetMirrorPos.vi"("error in (no error)"=w1037, "Mirror"=w1039, "Refnum In"=w1038) -> ("error out"=w1042:errorcluster, "Current Mirror Position"=w1036:i32, "Refnum Out"=w1041:refnum<k7>)  [unwired: 1 in]
                    n551 = local write "Entrance Mirror\nPosition"(w1036) -> ()
                    n552 = call "JYGetMirrorPos.vi"("error in (no error)"=w1042, "Mirror"=w1040, "Refnum In"=w1041) -> ("error out"=w1034:errorcluster, "Current Mirror Position"=w1035:i32)  [unwired: 1 in, 1 out]
                    n553 = local write "Exit Mirror\nPosition"(w1035) -> ()
                  }
                  frame #3 {
                    w1052 = u16 0 items=["Front Entrance", "Side Entrance", "Front Exit", "Side Exit", "First Intermediate", "Second Intermediate"] ("Slit")
                    # "Set New Slit Positions"
                    n554 = call "JYSlits.vi"("JYMONOLib.IJYMonoReqd"=w1054, "Slit"=w1052, "error in (no error)"=w1053, "Slit Width"="Target\nFront Entrance") -> ("error out"=w1050:errorcluster)  [unwired: 1 in, 1 out]
                  }
                }
              }
            }
          }
        }
        n555 = local read "Close"() -> (w992:bool)
      }
    }
  }
  n556 = flat-sequence {
    frame #0 {
      n557 = call <vilib>:"Create Report.vi"("window state (normal)"=T3."no change", "report type"=Report_Type."Excel", "template (empty)"=path "D:/desktop/train/TEST1/Save/2670中心波长.xlsx") -> ("report out"=w1061:refnum<class "NI_report.lvclass">, "error out"=w1060:errorcluster)  [unwired: 11 in]
      n558 = call-poly <vilib>:"Excel Get Data.vi"("report in"=w1061, "data type"=string[][] [], "error in (no error)"=w1060) -> ("report out"=w1056:refnum<class "NI_report.lvclass">, "data"=w1064:string[][], "error out"=w1055:errorcluster)  [unwired: 10 in]
      n559 = call-dynamic "Dispose Report.vi"("report in"=w1056, "error in (no error)"=w1055) -> ()  [unwired: 13 in, 1 out]
      n560 = Index Array(array=w1064, index (col)=0 ("禁用的索引 (列)")) -> (element=w1066:string[])  [unwired: 1 in]
      n561 = Fract/Exp String To Number(string=w1066) -> (number=→"波长范围":dbl[])  [unwired: 3 in, 1 out]
    }
  }
